vi "ME_acquire_21_HallSensor_LSchanB.vi"() -> ()   [LabVIEW 2015]
doc: "Use this template to build a producer/consumer design pattern. Use this template when you need to execute a process, such as data analysis, when a data source, such as a triggered acquisition, produces data at an uneven rate and you need to execute the process when the data becomes available."
uses:
  Mode.ctl
  oxford_driver/Oxford Drivers/BUSGEN.LLB/OxfordAddress.ctl
  <vilib>/Analysis/baseanly.llb/Mean (DBL).vi
  <vilib>/DAQmx/read.llb/DAQmx Read (Analog 1D DBL 1Chan NSamp).vi
  <vilib>/DAQmx/create/channels.llb/DAQmx Create Channel (AI-Voltage-Basic).vi
  <vilib>/DAQmx/configure/timing.llb/DAQmx Timing (Sample Clock).vi
  <vilib>/Utility/file.llb/Write Delimited Spreadsheet (DBL).vi
  <vilib>/DAQmx/miscellaneous.llb/DAQmx Fill In Error Info.vi
  <vilib>/express/express arith-compare/Formula/XNode/ExpressFormulaBlockNode.xnode
  <vilib>/Analysis/NI_AALBase.lvlib
panel:
  out "B lag":cluster{dbl[], dbl[]}(graph)
  out "T array":dbl[](array[numeric])
  out "Averaged I(T)":dbl[][](array[numeric])
  in  "Averaged P(T)":dbl[][](array[numeric])
  out "remaining elements 2":T1(array[cluster])
  out "Actual mean":dbl format="%0.6f"
  in  "Averaged dt":dbl[][](array[numeric])
  in  "Averaged P(B)":dbl[][](array[numeric])
  out "LockInR":dbl
  out "deltaUaux":dbl
  out "Hall Resistance (Ohm)":dbl caption="Actual AuxV" step=0.1
  in  "Stop":bool
  out "SaveSweep":bool=TRUE
  out "Measurement File_dn":path
  out "Measurement File_up":path
  out "Measurement File_average":path
  out "Actual Polarization":dbl
  in  "Reset IB?":bool
  in  "First?":bool
  in  "Save Period":dbl=1.0
  out "Averaged I(B)":dbl[][](array[numeric])
  out "P(uC/mm^2)":dbl[](array[numeric])
  in  "Sweep":bool
  out "Offset array":dbl[](array[numeric])
  in  "stop 2":bool
  in  "dB":dbl=0.005
  out "Actual B Field (T)":dbl
  out "Actual Temperature (K)":dbl
  out "Actual Current (pA)":dbl
  in  "Tab Control":T2(tab)
  in  "dt (K)":dbl=0.1
  in  "Max temperature (K)":dbl=20.0
  in  "Min Temperature (K)":dbl=4.5
  out "P(T)":cluster{"yi":dbl[], dbl[]}(graph)
  out "I(T)":cluster{dbl[], dbl[]}(graph)
  in  "Set temperature (K)":dbl=4.5
  in  "Temp Ramping Rate (K/min)":dbl=10.0
  in  "Heater Range":enum16{"Off", "Low", "Medium", "High"}(ring)
  in  "Heater On/Off":bool
  out "Setpoint Temperature (K)":dbl
  out "I(T) /Averaged/":cluster{"B array":dbl[], dbl[]}[](graph)
  out "P(T) /Averaged/":cluster{"B array":dbl[], dbl[]}[](graph)
  out "Up/Down 2":bool
  in  "Channel B/A":bool
  out "I(B) 3":cluster{dbl[], dbl[]}[](graph)
  out "I(B) /Averaged/":cluster{"B array":dbl[], dbl[]}[](graph)
  out "P(B) /Averaged/":cluster{"B array":dbl[], dbl[]}[](graph)
  out "P(B)":cluster{"yi":dbl[], dbl[]}(graph)
  in  "Set Field (T)":dbl
  in  "Go to Set":bool
  in  "Sweep Rate (T/min)":dbl=2.0 format="%.6f"
  in  "Field To Zero":bool
  out "Target Field":dbl
  in  "Min Field (T)":dbl
  in  "Max Field (T)":dbl=0.15
  in  "Threshold B (T)":dbl
  out "Up/Down":bool
  in  "Magnetic Field array (T)":dbl[](array[numeric])=[0.025, 0.05, 0.075, 0.1, 0.125, 0.15, 0.175, 0.2, 0.225, 0.25, 0.275, 0.3]
  in  "T Sweep Rate Array":dbl[](array[numeric])=[10.0, 20.0]
  in  "Max count array":i32[](array[numeric])=[2, 1, 0, 0, 0, 9, 10, 11, 12]
  in  "secs to wait":dbl=180.0
  out "Wait (s)":dbl
  in  "Directory":string
  out "Finished":bool=TRUE
  out "Step Rate":bool
  out "New":bool=TRUE
  in  "Temperature Array":dbl[](array[numeric])=[4.5, 5.0, 6.0, 7.0, 8.0, 9.0, 10.0, 11.0, 12.0]
  in  "Sweep Rate Array":dbl[](array[numeric])=[2.0, 1.0, 0.5, 0.1, 0.05, 9.0, 10.0, 11.0, 12.0]
  in  "Record ALL":bool
  in  "Max Countl":i32
  out "i":i32
  out "j":i32
  out "Step Temp":bool
  in  "FileName":string
  in  "Measure Noise":bool
  in  "Cycles":i32
  in  "maximum value":dbl=10.0 format="%0.2f"
  in  "minimum value":dbl=-10.0 format="%0.2f"
  in  "physical channels":tag="Dev1/ai1"
  out "PSD (pA/Hz^1/2) Peaks Removed":cluster{"f0":dbl, "df":dbl, "magnitude":dbl[]}(graph)
  out "PSD (pA/Hz^1/2)":cluster{"f0":dbl, "df":dbl, "magnitude":dbl[]}(graph)
  out "Current (pA) Filtered":waveform(dbl)(graph)
  out "Current (pA)":dbl[](graph)
  in  "Samples per channel":i32=1000
  in  "Rate":dbl=1000.0 format="%0.2f"
  in  "Cut-Off Frequency":dbl=100.0 caption="Lower Cut-Off"
  in  "Filter On":bool
  in  "Keithley (IV conv) averaging":i32=10
  in  "Lock_in_Amplifier":refnum<visa-resource-name>="GPIB0::5::INSTR"
  out "Dc offset":dbl
  in  "Calibrate":bool
  in  "IV converter":refnum<visa-resource-name>="GPIB0::20::INSTR"
  in  "Magnetic Field":refnum<visa-resource-name>="GPIB0::19::INSTR"
  out "Time Lag":dbl=0.0500025749206543
  in  "Lake Shore":refnum<visa-resource-name>="GPIB0::11::INSTR"
  in  "Temp Refresh (s)":dbl=0.1
  in  "Sampling rate (Hz)":dbl=10.0
  in  "Gain (V/A)":dbl=1000000000.0
  in  "Sample area (mm^2)":dbl=1.0
  out "Calibration Curve":cluster{dbl[], "Best Linear Fit":dbl[]}[](graph)=[{[0.0, 0.005, 0.01, 0.015, 0.02, 0.025, 0.03, 0.035, 0.04, 0.045, 0.05, 0.055, 0.06, 0.065, 0.07, 0.075, 0.08, 0.085, 0.09, 0.095, 0.1, 0.105, 0.11, 0.115, 0.12, 0.125, 0.13, 0.135, 0.14, 0.145, 0.15, 0.155, 0.16, 0.165, 0.17, 0.175, 0.18, 0.185, 0.19, 0.195, 0.2, 0.205, 0.21, 0.215, 0.22, 0.225, 0.23, 0.235, 0.24, 0.245, 0.25, 0.255, 0.26, 0.265, 0.27, 0.275, 0.28, 0.285, 0.29, 0.295, 0.3, 0.305, 0.31, 0.315, 0.32, 0.325, 0.33, 0.335, 0.34, 0.345, 0.35, 0.355, 0.36, 0.365, 0.37, 0.375, 0.38, 0.385, 0.39, 0.395, 0.4, 0.405, 0.41, 0.415, 0.42, 0.425, 0.43, 0.435, 0.44, 0.445, 0.45, 0.455, 0.46, 0.465, 0.47, 0.475, 0.48, 0.485, 0.49, 0.495, 0.5], "Best Linear Fit"=[-1.7e-06, 1.18e-05, 3.66e-05, 6.17e-05, 9.39e-05, 0.000122, 0.0001511, 0.0001781, 0.0002061, 0.0002355, 0.0002616, 0.0002895, 0.0003184, 0.0003446, 0.0003689, 0.0003958, 0.0004207, 0.0004464, 0.0004684, 0.0004953, 0.0005218, 0.0005459, 0.0005692, 0.0005897, 0.0006131, 0.0006347, 0.0006589, 0.0006834, 0.0007035, 0.0007249, 0.0007465, 0.000765, 0.0007858, 0.0008103, 0.0008302, 0.0008467, 0.000868, 0.0008855, 0.0009079, 0.0009248, 0.0009452, 0.0009633, 0.0009828, 0.0009992, 0.0010189, 0.0010338, 0.001054, 0.0010692, 0.0010858, 0.0011036, 0.0011162, 0.0011356, 0.0011502, 0.0011643, 0.0011834, 0.0011985, 0.0012131, 0.0012277, 0.0012423, 0.0012571, 0.0012691, 0.0012827, 0.0012976, 0.001313, 0.0013264, 0.0013388, 0.0013518, 0.0013638, 0.0013782, 0.0013909, 0.0014035, 0.0014175, 0.0014295, 0.0014407, 0.0014538, 0.0014641, 0.0014752, 0.0014861, 0.0014978, 0.0015081, 0.0015203, 0.001532, 0.0015422, 0.0015526, 0.001563, 0.0015754, 0.0015844, 0.0015955, 0.0016056, 0.001614, 0.0016239, 0.0016342, 0.0016457, 0.0016542, 0.0016635, 0.001674, 0.001681, 0.0016886, 0.0016986, 0.0017063, 0.0017155]}, {[0.0, 0.005, 0.01, 0.015, 0.02, 0.025, 0.03, 0.035, 0.04, 0.045, 0.05, 0.055, 0.06, 0.065, 0.07, 0.075, 0.08, 0.085, 0.09, 0.095, 0.1, 0.105, 0.11, 0.115, 0.12, 0.125, 0.13, 0.135, 0.14, 0.145, 0.15, 0.155, 0.16, 0.165, 0.17, 0.175, 0.18, 0.185, 0.19, 0.195, 0.2, 0.205, 0.21, 0.215, 0.22, 0.225, 0.23, 0.235, 0.24, 0.245, 0.25, 0.255, 0.26, 0.265, 0.27, 0.275, 0.28, 0.285, 0.29, 0.295, 0.3, 0.305, 0.31, 0.315, 0.32, 0.325, 0.33, 0.335, 0.34, 0.345, 0.35, 0.355, 0.36, 0.365, 0.37, 0.375, 0.38, 0.385, 0.39, 0.395, 0.4, 0.405, 0.41, 0.415, 0.42, 0.425, 0.43, 0.435, 0.44, 0.445, 0.45, 0.455, 0.46, 0.465, 0.47, 0.475, 0.48, 0.485, 0.49, 0.495, 0.5], "Best Linear Fit"=[-1.7e-06, 1.18e-05, 3.66e-05, 6.17e-05, 9.39e-05, 0.000122, 0.0001511, 0.0001781, 0.0002061, 0.0002355, 0.0002616, 0.0002895, 0.0003184, 0.0003446, 0.0003689, 0.0003958, 0.0004207, 0.0004464, 0.0004684, 0.0004953, 0.0005218, 0.0005459, 0.0005692, 0.0005897, 0.0006131, 0.0006347, 0.0006589, 0.0006834, 0.0007035, 0.0007249, 0.0007465, 0.000765, 0.0007858, 0.0008103, 0.0008302, 0.0008467, 0.000868, 0.0008855, 0.0009079, 0.0009248, 0.0009452, 0.0009633, 0.0009828, 0.0009992, 0.0010189, 0.0010338, 0.001054, 0.0010692, 0.0010858, 0.0011036, 0.0011162, 0.0011356, 0.0011502, 0.0011643, 0.0011834, 0.0011985, 0.0012131, 0.0012277, 0.0012423, 0.0012571, 0.0012691, 0.0012827, 0.0012976, 0.001313, 0.0013264, 0.0013388, 0.0013518, 0.0013638, 0.0013782, 0.0013909, 0.0014035, 0.0014175, 0.0014295, 0.0014407, 0.0014538, 0.0014641, 0.0014752, 0.0014861, 0.0014978, 0.0015081, 0.0015203, 0.001532, 0.0015422, 0.0015526, 0.001563, 0.0015754, 0.0015844, 0.0015955, 0.0016056, 0.001614, 0.0016239, 0.0016342, 0.0016457, 0.0016542, 0.0016635, 0.001674, 0.001681, 0.0016886, 0.0016986, 0.0017063, 0.0017155]}]
  in  "Offset?":bool
  in  "Magnet":bool=TRUE
  in  "Ramp":bool=TRUE
  in  "DaQ":bool
  in  "Moving average":i8=10
  in  "Sample Rate":dbl=1000.0
  in  "Number of Samples":i32=100
  in  "Physical Channel":tag="kartya/ai0"
  in  "Min Voltage":dbl=-5.0
  in  "Max Voltage":dbl=5.0
  in  "Terminal Configuration":i32(ring)=-1 items=["default"=-1, "RSE"=10083, "NRSE"=10078, "Differential"=10106, "Pseudodifferential"=12529]
  out "Confirm":bool
  in  "Dwell Time (ms)":u32=1000
  out "Calibration Curve Data":dbl[][](array[numeric])=[[0.0, 0.005, 0.01, 0.015, 0.02, 0.025, 0.03, 0.035, 0.04, 0.045, 0.05, 0.055, 0.06, 0.065, 0.07, 0.075, 0.08, 0.085, 0.09, 0.095, 0.1, 0.105, 0.11, 0.115, 0.12, 0.125, 0.13, 0.135, 0.14, 0.145, 0.15, 0.155, 0.16, 0.165, 0.17, 0.175, 0.18, 0.185, 0.19, 0.195, 0.2, 0.205, 0.21, 0.215, 0.22, 0.225, 0.23, 0.235, 0.24, 0.245, 0.25, 0.255, 0.26, 0.265, 0.27, 0.275, 0.28, 0.285, 0.29, 0.295, 0.3, 0.305, 0.31, 0.315, 0.32, 0.325, 0.33, 0.335, 0.34, 0.345, 0.35, 0.355, 0.36, 0.365, 0.37, 0.375, 0.38, 0.385, 0.39, 0.395, 0.4, 0.405, 0.41, 0.415, 0.42, 0.425, 0.43, 0.435, 0.44, 0.445, 0.45, 0.455, 0.46, 0.465, 0.47, 0.475, 0.48, 0.485, 0.49, 0.495, 0.5], [-1.7e-06, 1.18e-05, 3.66e-05, 6.17e-05, 9.39e-05, 0.000122, 0.0001511, 0.0001781, 0.0002061, 0.0002355, 0.0002616, 0.0002895, 0.0003184, 0.0003446, 0.0003689, 0.0003958, 0.0004207, 0.0004464, 0.0004684, 0.0004953, 0.0005218, 0.0005459, 0.0005692, 0.0005897, 0.0006131, 0.0006347, 0.0006589, 0.0006834, 0.0007035, 0.0007249, 0.0007465, 0.000765, 0.0007858, 0.0008103, 0.0008302, 0.0008467, 0.000868, 0.0008855, 0.0009079, 0.0009248, 0.0009452, 0.0009633, 0.0009828, 0.0009992, 0.0010189, 0.0010338, 0.001054, 0.0010692, 0.0010858, 0.0011036, 0.0011162, 0.0011356, 0.0011502, 0.0011643, 0.0011834, 0.0011985, 0.0012131, 0.0012277, 0.0012423, 0.0012571, 0.0012691, 0.0012827, 0.0012976, 0.001313, 0.0013264, 0.0013388, 0.0013518, 0.0013638, 0.0013782, 0.0013909, 0.0014035, 0.0014175, 0.0014295, 0.0014407, 0.0014538, 0.0014641, 0.0014752, 0.0014861, 0.0014978, 0.0015081, 0.0015203, 0.001532, 0.0015422, 0.0015526, 0.001563, 0.0015754, 0.0015844, 0.0015955, 0.0016056, 0.001614, 0.0016239, 0.0016342, 0.0016457, 0.0016542, 0.0016635, 0.001674, 0.001681, 0.0016886, 0.0016986, 0.0017063, 0.0017155]]
  in  "Start Field":dbl
  in  "Max Field":dbl=0.5 format="%#_13g"
  in  "Temp/Magnetic Field":bool
  out "index":i8
  out "Read?":bool
  out "Magnetic Field (T)":dbl[](array[numeric])
  out "Reset":bool
  out "Measured Current (pA)":dbl[](array[numeric])
  out "Elapsed Time (s)":dbl[](array[numeric])
  out "Start time":timestamp
  in  "Enum":T3=enum."Process"
  out "B array":dbl[](array[numeric])
  in  "dB (T)":dbl=0.0025
  in  "Counter":i8
  out "L magnet (H)":dbl
  out "R magnet (mOhm)":dbl
  out "Actual Current (R0)":dbl
  out "Nominal Field (T)":dbl
  out "Temperature array":dbl[](array[numeric])
  in  "New Measurement File":bool
  out "Measurement File":path
  out "refnum out":refnum<file>
  in  "Measuring":bool
  in  "Measure /Pause":bool
  in  "stop":bool
  # "DeltaForce"
  # "Discrete"
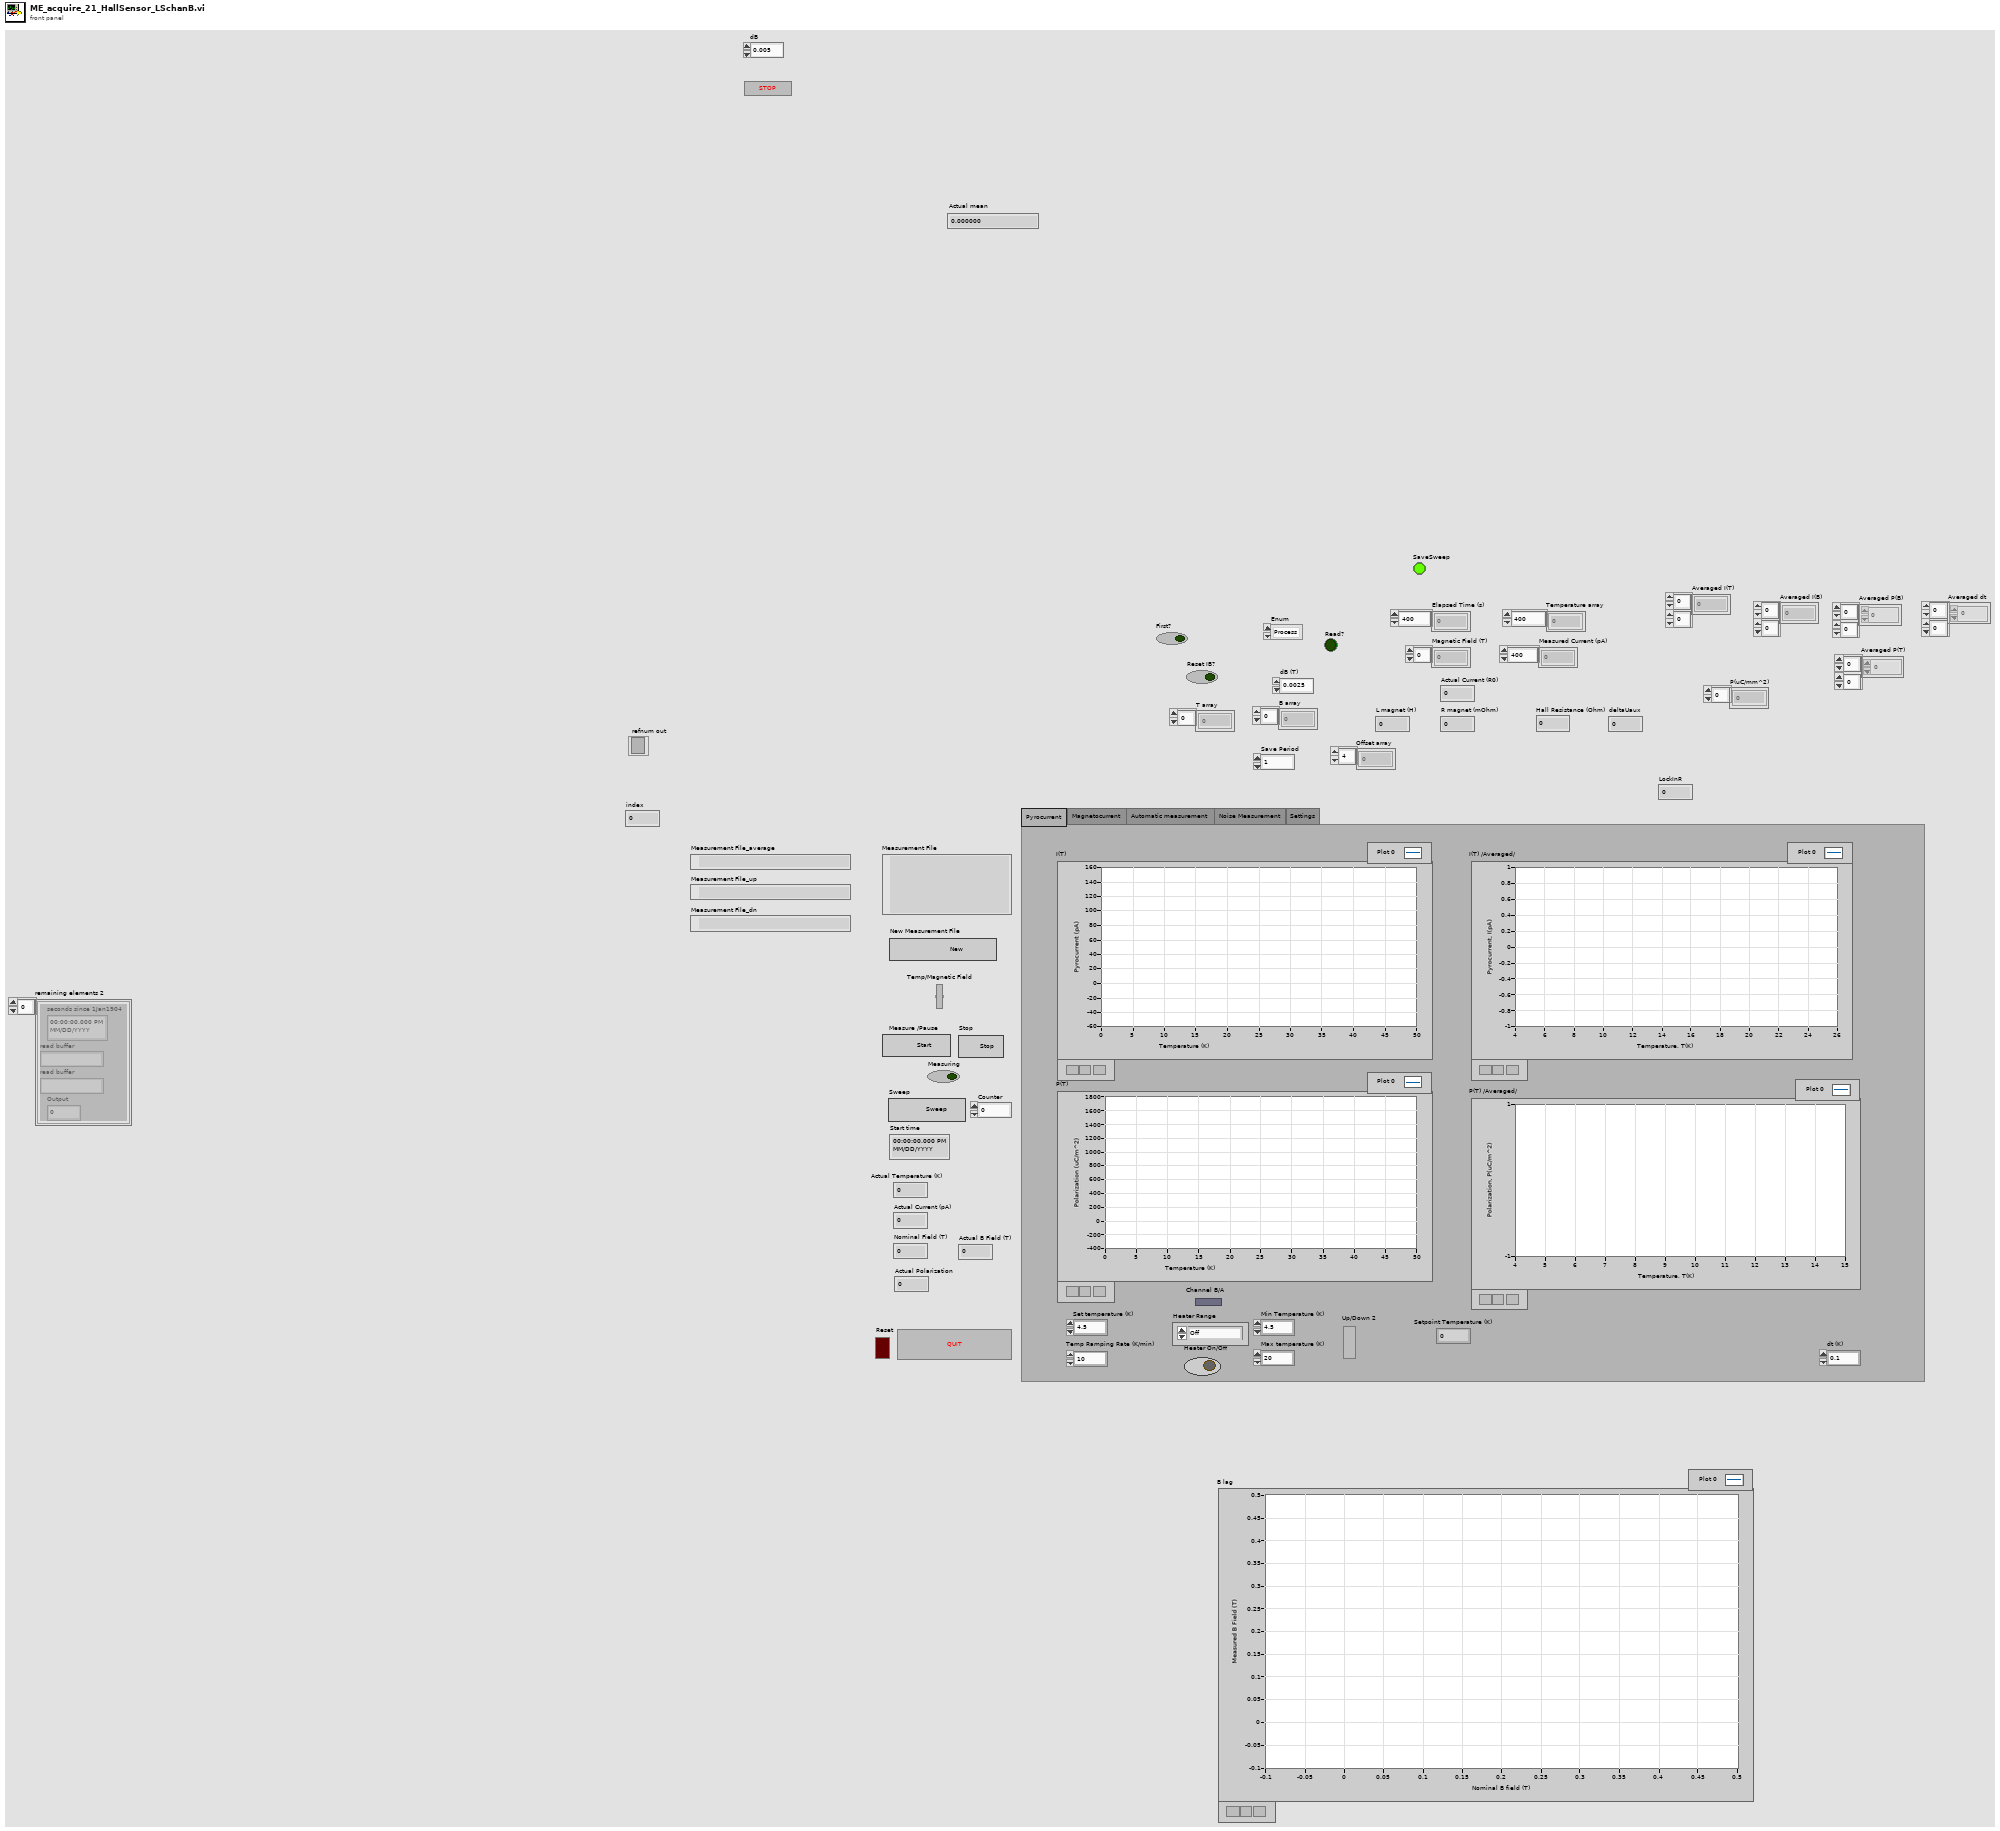
[diagram p1: front panel]
types:
  T1 = cluster{"seconds since 1Jan1904":timestamp, "read buffer":string, "read buffer":string, "Output":dbl}[]
  T2 = enum32{"Pyrocurrent", "Magnetocurrent", "Automatic measurement", "Noise Measurement", "Settings"}
  T3 = typedef "Mode.ctl" = enum16{"Offset", "Process", "Sweep", "StepOxford", "StepDelta", "Plot", "Save", "New", "Return", ""}
  T4 = cluster{"seconds since 1Jan1904":timestamp, "read buffer":string, "read buffer":string, "Output":dbl}
  T5 = enum16{"open", "replace", "create", "open or create", "replace or create", "replace or create with confirmation"}
  T6 = typedef "OxfordAddress.ctl" = cluster{"Com Port":i32, "ISOBUS Address":i32, "GPIB Address":i16, "Communication":enum16{"RS232", "ISOBUS", "GPIB", "Gateway"}}
  T7 = cluster{"B array":dbl[], "Averaged P(B) Out":dbl[]}
  T8 = cluster{"B array":dbl[], "BaselineSubtracted I(B)":dbl[]}
  T9 = cluster{"B array":dbl[], "Averaged P(B) Out":dbl[]}[]
  T10 = cluster{"B array":dbl[], "BaselineSubtracted I(B)":dbl[]}[]
  T11 = cluster{"T array":dbl[], "Averaged P(T) Out":dbl[]}
  T12 = cluster{"T array":dbl[], "Averaged I(B) out":dbl[]}
  T13 = cluster{"T array":dbl[], "Averaged P(T) Out":dbl[]}[]
  T14 = cluster{"T array":dbl[], "Averaged I(B) out":dbl[]}[]
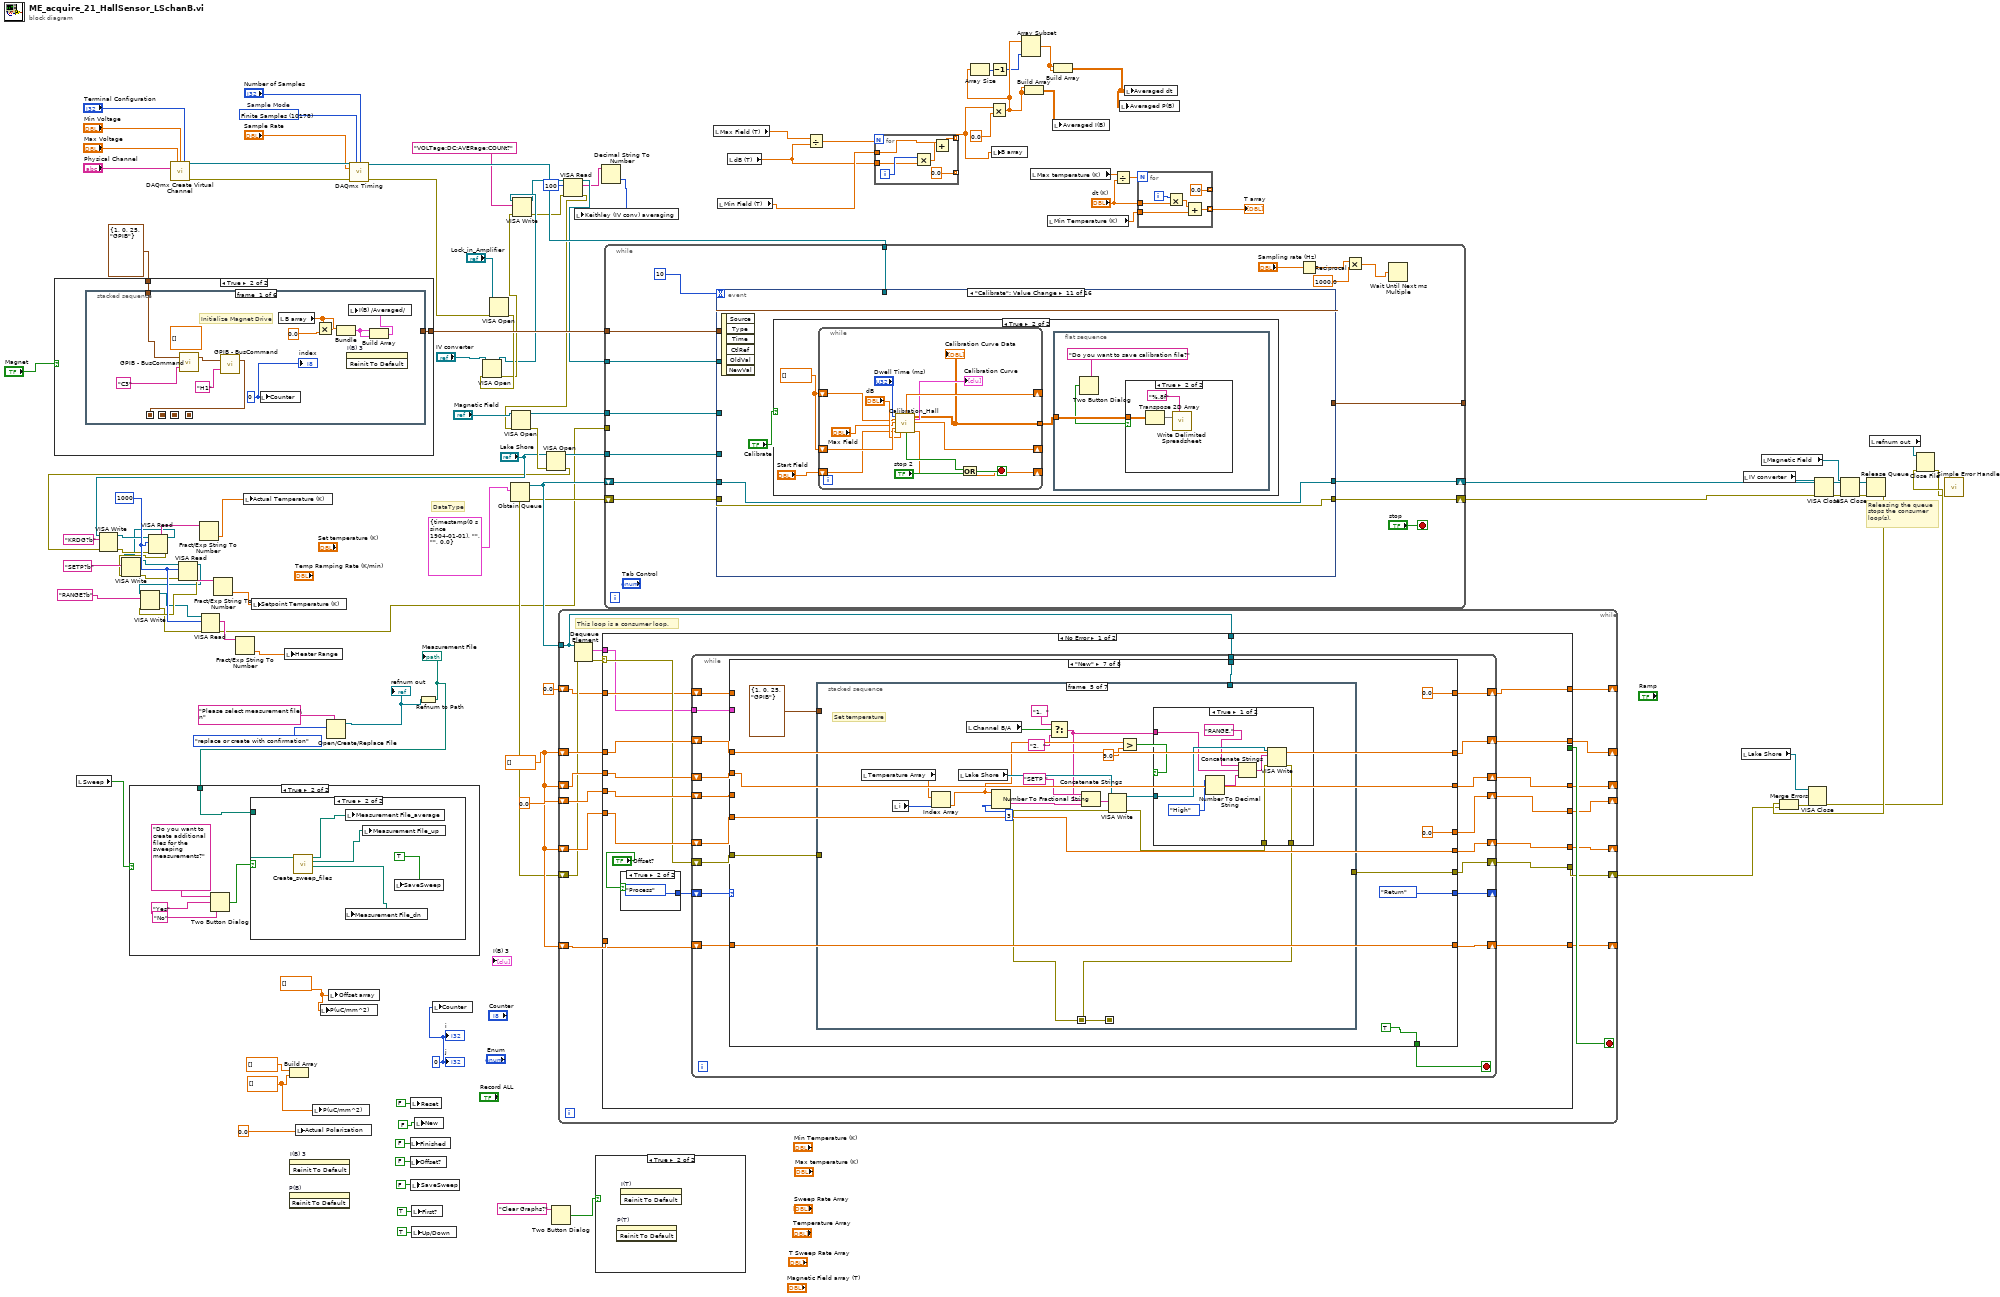
[diagram p0: block diagram]
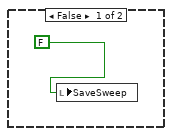
[diagram p4: hidden frame]
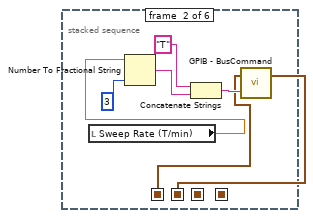
[diagram p6: hidden frame]
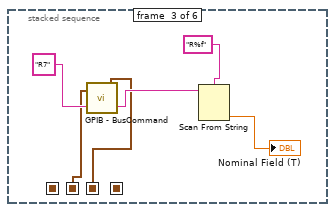
[diagram p7: hidden frame]
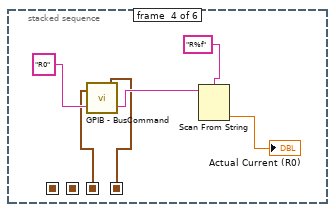
[diagram p8: hidden frame]
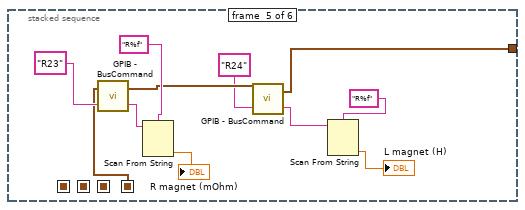
[diagram p9: hidden frame]
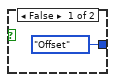
[diagram p11: hidden frame]
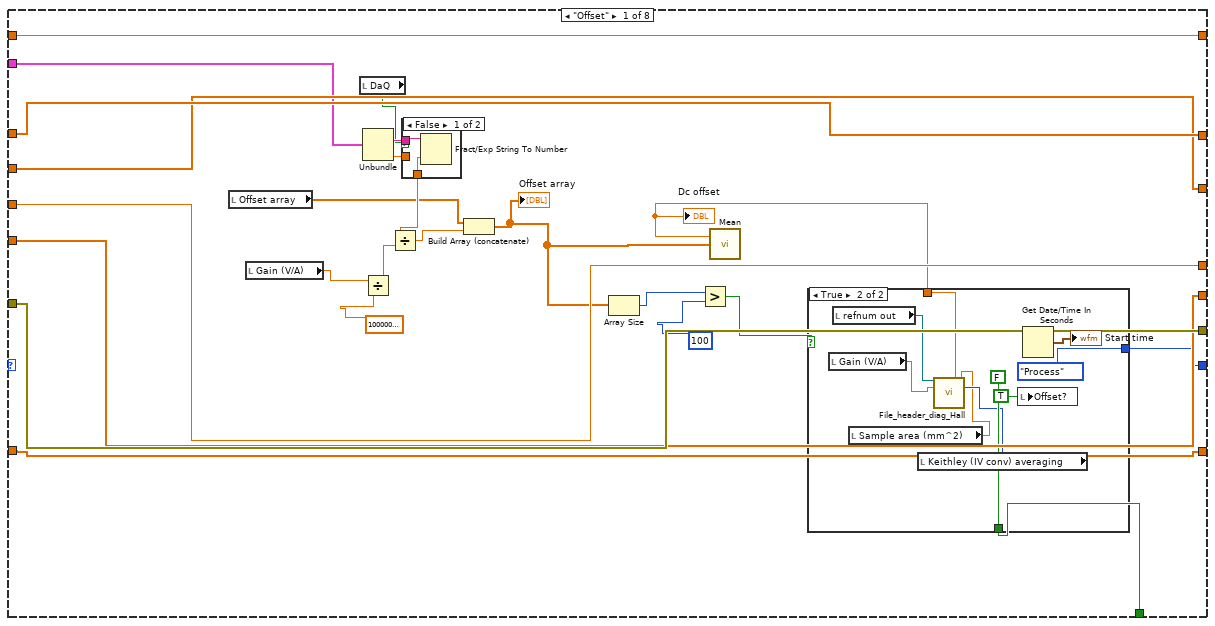
[diagram p12: hidden frame]
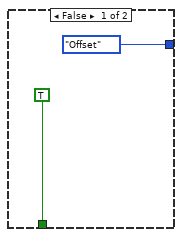
[diagram p14: hidden frame]
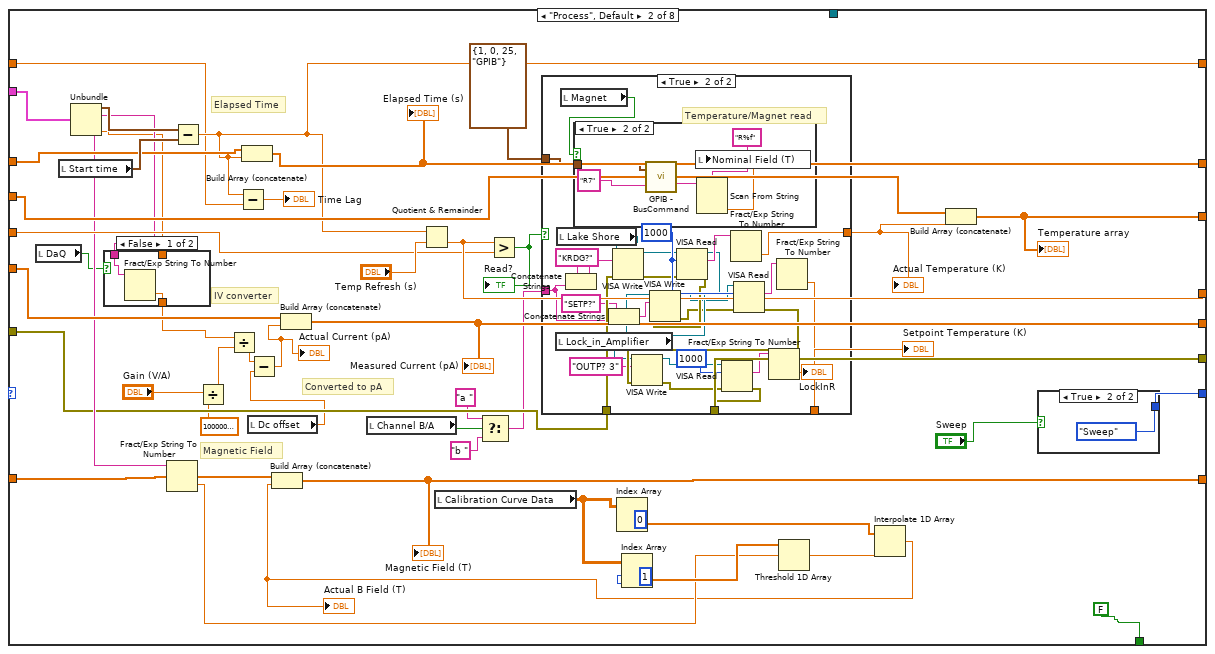
[diagram p15: hidden frame]
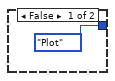
[diagram p17: hidden frame]
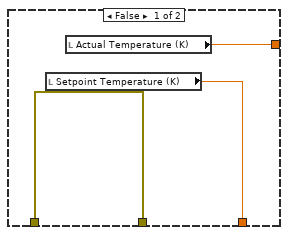
[diagram p18: hidden frame]
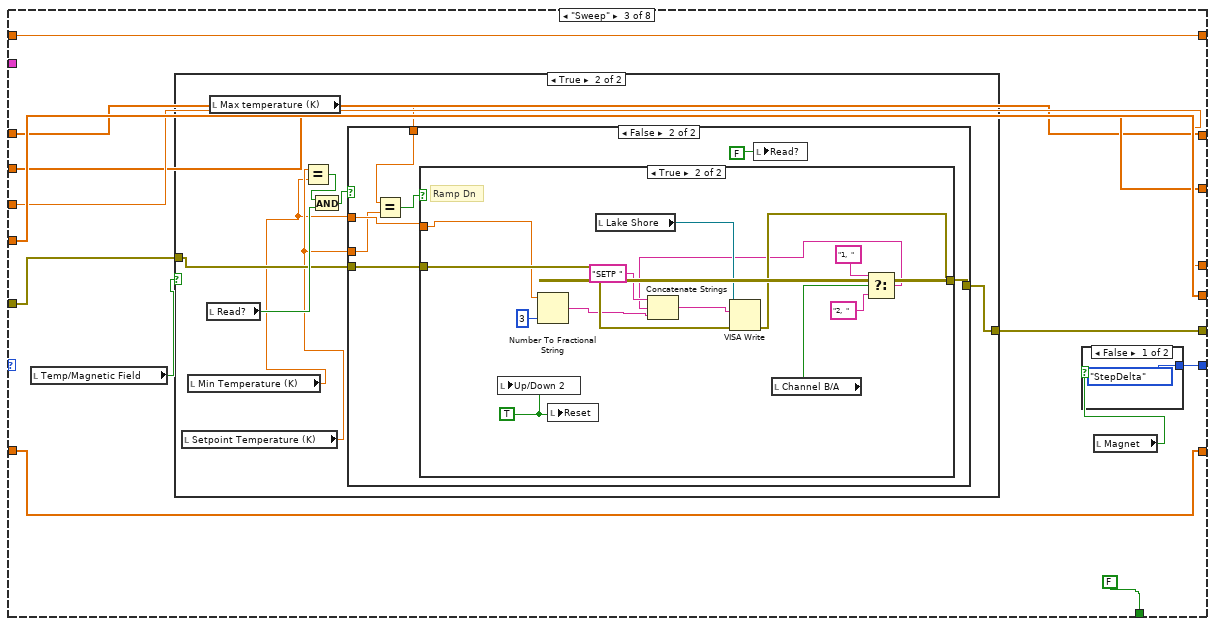
[diagram p20: hidden frame]
diagram:
  w27 = 10178 items=["Finite Samples"=10178, "Continuous Samples"=10123, "Hardware Timed Single Point"=12522]  # Sample Mode
  w54 = u32 1000 ("byte count")
  w65 = 0 ("j")
  w62 = dbl[] []
  w80 = dbl[] []
  w86 = dbl[] []
  # "DataType"
  # "Releasing the queue stops the consumer loop(s)."
  n1 = case shown="True" "Magnet" {
    tunnel: T6 {"Com Port"=1, "ISOBUS Address"=0, "GPIB Address"=25, "Communication"=enum."GPIB"} ("Address") -> [w110 w112]
    tunnel: [w110 w111] -> w92
    frame False {
    }
    frame True {
      n2 = stacked-sequence {
        seq-local: [w120 _ _ _ _ _] -> [_ w125 _ _ _ _]
        seq-local: [_ w124 _ _ _ _] -> [_ _ w132 _ _ _]
        seq-local: [_ _ w131 _ _ _] -> [_ _ _ w138 _ _]
        seq-local: [_ _ _ w137 _ _] -> [_ _ _ _ w149 _]
        tunnel: w112 -> [w122 _ _ _ _ _]
        tunnel: [_ _ _ _ w147 _] -> w111
        frame #0 {
          (unwired) dbl[][] []
          w118 = i8 0 ("Counter")
          # "Initialize Magnet Drive"
          n3 = call "GPIB - BusCommand.vi"("Command"="C3", "Address"=w122) -> ("Address(thru)"=w121:T6)  [unwired: 1 out]
          n4 = call "GPIB - BusCommand.vi"("Command"="H1", "Address"=w121) -> ("Address(thru)"=w120:T6)  [unwired: 1 out]
          n5 = local write "Counter"(w118) -> ()
          n6 = local read "B array"() -> (w116:dbl[])
          n7 = Multiply(x=w116, y=0.0) -> (x*y=w115:dbl[])
          n8 = Bundle("B array"=w116, w115) -> (w114:cluster{"B array":dbl[], dbl[]})  [unwired: 1 in]
          n9 = invoke on="I(B) 3" class="XYGraph (strict)" method="Reinit To Default"() -> ()  [unwired: 3 in, 3 out]
          n10 = Build Array(w114, w114) -> (w113:cluster{"B array":dbl[], dbl[]}[])
          n11 = local write "I(B) /Averaged/"(w113) -> ()
          "index" <- w118
        }
        frame #1 {
          n12 = local read "Sweep Rate (T/min)"() -> (w126:dbl)
          n13 = Number To Fractional String(number=w126, precision (6)=i16 3) -> (F-format string=w128:string)  [unwired: 2 in]
          n14 = Concatenate Strings("T" ("format string"), w128) -> (w127:string)
          n15 = call "GPIB - BusCommand.vi"("Command"=w127, "Address"=w125) -> ("Address(thru)"=w124:T6)  [unwired: 1 out]
        }
        frame #2 {
          n16 = call "GPIB - BusCommand.vi"("Command"="R7" ("format string"), "Address"=w132) -> ("Reply"=w136:string, "Address(thru)"=w131:T6)
          n17 = Scan From String(format string="R%f" ("remaining string"), input string=w136) -> (output 1=→"Nominal Field (T)":dbl)  [unwired: 3 in, 3 out]
        }
        frame #3 {
          n18 = call "GPIB - BusCommand.vi"("Command"="R0" ("format string"), "Address"=w138) -> ("Reply"=w142:string, "Address(thru)"=w137:T6)
          n19 = Scan From String(format string="R%f" ("remaining string"), input string=w142) -> (output 1=→"Actual Current (R0)":dbl)  [unwired: 3 in, 3 out]
        }
        frame #4 {
          n20 = call "GPIB - BusCommand.vi"("Command"="R23" ("format string"), "Address"=w149) -> ("Reply"=w153:string, "Address(thru)"=w148:T6)
          n21 = Scan From String(format string="R%f" ("remaining string"), input string=w153) -> (output 1=→"R magnet (mOhm)":dbl)  [unwired: 3 in, 3 out]
          n22 = call "GPIB - BusCommand.vi"("Command"="R24" ("format string"), "Address"=w148) -> ("Reply"=w145:string, "Address(thru)"=w147:T6)
          n23 = Scan From String(format string="R%f" ("remaining string"), input string=w145) -> (output 1=→"L magnet (H)":dbl)  [unwired: 3 in, 3 out]
        }
        frame #5 {
        }
      }
    }
  }
  n24 = local read "Sweep"() -> (w70:bool)
  n25 = call-poly <vilib>:"DAQmx Create Virtual Channel.vi"("maximum value"="Max Voltage", "minimum value"="Min Voltage", "input terminal configuration"="Terminal Configuration", "physical channels"="Physical Channel") -> ("task out"=w25:refnum<k21>, "error out"=w26:errorcluster)  [unwired: 10 in]
  n26 = Build Array(dbl[] [], w62) -> ()  [unwired: 1 out]
  n27 = invoke on="P(B)" class="XYGraph (strict)" method="Reinit To Default"() -> ()  [unwired: 3 in, 3 out]
  n28 = invoke on="I(B) 3" class="XYGraph (strict)" method="Reinit To Default"() -> ()  [unwired: 3 in, 3 out]
  n29 = local write "Actual Polarization"(0.0 ("Actual Polarization")) -> ()
  n30 = local write "P(uC/mm^2)"(w62) -> ()
  n31 = local write "P(uC/mm^2)"(w80) -> ()
  n32 = Open/Create/Replace File(prompt="Please select measurement file\n", operation (0:open)=T5."replace or create with confirmation") -> (refnum out=w89:refnum<file>)  [unwired: 4 in, 2 out]
  "refnum out" <- w89
  n33 = local write "Offset array"(w80) -> ()
  n34 = call-poly <vilib>:"DAQmx Timing.vi"("task/channels in"=w25, "sample mode"=w27, "samples per channel"="Number of Samples", "rate"="Sample Rate", "error in"=w26) -> ("task out"=w17:refnum<k21>, "error out"=w18:errorcluster)  [unwired: 9 in]
  n35 = local write "Finished"(FALSE ("Finished")) -> ()
  n36 = local write "Offset?"(FALSE ("Offset?")) -> ()
  n37 = local write "Reset"(FALSE ("Reset")) -> ()
  n38 = local write "SaveSweep"(FALSE ("SaveSweep")) -> ()
  n39 = local write "First?"(TRUE ("First?")) -> ()
  n40 = local write "Up/Down"(TRUE ("Up/Down")) -> ()
  n41 = local write "New"(FALSE ("New")) -> ()
  n42 = Refnum to Path(1:w89) -> (0:w69:path)
  "Measurement File" <- w69
  n43 = case shown="True" w70 {
    tunnel: w69 -> [_ w154]
    frame False {
    }
    frame True {
      n44 = Two Button Dialog(message="Do you want to create additional files for the sweeping measurements?" ("string"), 1:"No" ("F button name (\"Cancel\")"), 2:"Yes" ("T button name (\"OK\")")) -> (T button?=w156:bool)
      n45 = case shown="True" w156 {
        tunnel: w154 -> [_ w164]
        frame False {
          n46 = local write "SaveSweep"(FALSE ("SaveSweep")) -> ()
        }
        frame True {
          n47 = call "Create_sweep_files.vi"("Measurement File"=w164) -> ("Path 3"=w161:path, "Path 2"=w162:path, "Path"=w163:path)  [unwired: 8 in]
          n48 = local write "Measurement File_dn"(w161) -> ()
          n49 = local write "Measurement File_average"(w163) -> ()
          n50 = local write "Measurement File_up"(w162) -> ()
          n51 = local write "SaveSweep"(TRUE) -> ()
        }
      }
    }
  }
  n52 = local write "Counter"(w65) -> ()
  n53 = VISA Open(error in (no error)=w18, VISA resource name="Lock_in_Amplifier") -> (error out=w37:errorcluster)  [unwired: 3 in, 1 out]
  n54 = VISA Open(error in (no error)=w37, VISA resource name="IV converter") -> (VISA resource name=w14:refnum<visa-resource-name>, error out=w15:errorcluster)  [unwired: 3 in]
  n55 = Obtain Queue(element data type=T4 {"seconds since 1Jan1904"=timestamp(0 s since 1904-01-01), "read buffer"="", "read buffer"="", "Output"=0.0} ("output cluster")) -> (queue out=w109:refnum<queue>, error out=w84:errorcluster)  [unwired: 4 in, 1 out]
  n56 = VISA Write(VISA resource name=w14, write buffer="VOLTage:DC:AVERage:COUNt?", error in (no error)=w15) -> (VISA resource name out=w10:refnum<visa-resource-name>, error out=w12:errorcluster)  [unwired: 1 out]
  n57 = Two Button Dialog(message="Clear Graphs?") -> (T button?=w64:bool)  [unwired: 2 in]
  n58 = while {
    tunnel: w109 -> [w165]
    shift-right: [w178] -> _
    shift-left: w86 -> [w177]
    shift-right: [w176] -> _
    shift-left: w86 -> [w175]
    shift-right: [w174] -> _
    shift-left: w86 -> [w173]
    shift-right: [w172] -> _
    shift-left: 0.0 -> [w171]
    shift-right: [w170] -> _
    shift-left: w86 -> [w169]
    shift-right: [w179] -> w97
    shift-left: w84 -> [w168]
    shift-right: [w167] -> _
    shift-left: 0.0 -> [w166]
    stop <- w180 stop-if-true
    # "This loop is a consumer loop."
    n59 = Dequeue Element(queue=w165, error in (no error)=w168) -> (element=w181:T4, error out=w182:errorcluster)  [unwired: 1 in, 2 out]
    n60 = case shown="No Error" w182 {
      selector: w182 -> [w189 w956]
      tunnel: w181 -> [w183 _]
      tunnel: [_ TRUE] -> w180
      tunnel: [w188 w956] -> w179
      tunnel: [w199 w955] -> w178
      tunnel: w177 -> [w198 w955]
      tunnel: [w197 w952] -> w176
      tunnel: w175 -> [w196 w952]
      tunnel: [w195 w951] -> w174
      tunnel: w173 -> [w194 w951]
      tunnel: [w193 w953] -> w172
      tunnel: w171 -> [w192 w953]
      tunnel: [w191 w954] -> w170
      tunnel: w169 -> [w190 w954]
      tunnel: [w187 w950] -> w167
      tunnel: w166 -> [w186 w950]
      tunnel: w165 -> [w184 _]
      frame No Error {
        n61 = case shown="True" "Offset?" {
          tunnel: [Mode."Offset" ("Enum") Mode."Process" ("Enum")] -> w200
          frame False {
          }
          frame True {
          }
        }
        n62 = while {
          shift-right: [w209] -> _
          shift-left: w200 -> [w221]
          tunnel: w183 -> [w220]
          shift-right: [w219] -> w199
          shift-left: w198 -> [w218]
          shift-right: [w211] -> w191
          shift-left: w190 -> [w210]
          shift-right: [w213] -> w193
          shift-left: w192 -> [w212]
          shift-right: [w217] -> w197
          shift-left: w196 -> [w216]
          shift-right: [w207] -> w188
          shift-left: w189 -> [w208]
          shift-right: [w215] -> w195
          shift-left: w194 -> [w214]
          shift-right: [w205] -> w187
          shift-left: w186 -> [w204]
          tunnel: w184 -> [w203]
          stop <- w206 stop-if-true
          n63 = case shown="\"New\"" w221 {
            selector: w221 -> [_ _ _ _ _ _ _ w943]
            tunnel: w220 -> [w239 w306 _ _ _ _ _ _]
            tunnel: [w245 w303 w355 w497 w553 w626 w739 w948] -> w219
            tunnel: w218 -> [w245 w298 w355 w497 w553 w622 w739 w948]
            tunnel: [w240 w302 w358 w494 w555 w628 w737 w945] -> w217
            tunnel: w216 -> [w240 w301 w358 w494 w555 w623 w737 w945]
            tunnel: [w241 w300 w360 w492 w550 w629 w735 w942] -> w215
            tunnel: w214 -> [w241 w299 w360 w492 w550 w624 w735 w942]
            tunnel: [w243 w297 w357 w495 w551 w632 0.0 w946] -> w213
            tunnel: w212 -> [w243 w296 w357 w495 w551 w632 _ w946]
            tunnel: [w244 w293 w356 w496 w552 w627 w738 w947] -> w211
            tunnel: w210 -> [w244 w294 w356 w496 w552 w625 w738 w947]
            tunnel: [w228 w291 w353 Mode."Plot" ("Enum") Mode."Save" ("Enum") w633 Mode."Return" ("Enum") w943] -> w209
            tunnel: w208 -> [w242 w289 w362 w489 w558 w631 w731 w944]
            tunnel: [w242 w288 w361 w488 w558 w631 w730 w944] -> w207
            tunnel: [w224 FALSE FALSE FALSE FALSE w620 TRUE TRUE] -> w206
            tunnel: [w227 w285 w354 w490 w554 w630 0.0 w949] -> w205
            tunnel: w204 -> [w227 w284 w354 w490 w554 w630 _ w949]
            tunnel: w203 -> [_ _ _ _ _ _ w729 _]
            frame "Offset" {
              n64 = local read "Offset array"() -> (w233:dbl[])
              n65 = local read "Gain (V/A)"() -> (w237:dbl)
              n66 = local read "DaQ"() -> (w223:bool)
              n67 = Unbundle(w239) -> ("read buffer"=w226:string, "Output"=w222:dbl)  [unwired: 2 out]
              n68 = Divide(x=w237, y=1000000000000.0) -> (x/y=w235:dbl)
              n69 = case shown="False" w223 {
                tunnel: [w247 w248] -> w238
                tunnel: w226 -> [w246 _]
                tunnel: w222 -> [_ w248]
                frame False {
                  n70 = Fract/Exp String To Number(string=w246) -> (number=w247:dbl)  [unwired: 3 in, 1 out]
                }
                frame True {
                }
              }
              n71 = Divide(x=w238, y=w235) -> (x/y=w234:dbl)
              n72 = Build Array (concatenate)(w233, w234) -> (w229:dbl[])
              "Offset array" <- w229
              n73 = Array Size(array=w229) -> (size(s)=w232:i32)
              n74 = Greater?(x=w232, y=100) -> (0:w230:bool)
              n75 = call-poly <vilib>:"Mean.vi"("X"=w229) -> ("mean"=w225:dbl)  [unwired: 1 out]
              "Dc offset" <- w225
              n76 = case shown="True" w230 {
                tunnel: [Mode."Offset" ("Enum") Mode."Process" ("Enum")] -> w228
                tunnel: w225 -> [_ w255]
                tunnel: [TRUE FALSE] -> w224
                frame False {
                }
                frame True {
                  n77 = local read "Gain (V/A)"() -> (w256:dbl)
                  n78 = local read "refnum out"() -> (w257:refnum<file>)
                  n79 = local read "Sample area (mm^2)"() -> (w251:dbl)
                  n80 = local read "Keithley (IV conv) averaging"() -> (w252:i32)
                  n81 = call "File_header_diag_Hall.vi"("Byte Stream File in"=w257, "OFFSET"=w255, "Sample area"=w251, "Gain"=w256, "Averaging"=w252) -> ()  [unwired: 11 in]
                  n82 = local write "Offset?"(TRUE ("Offset?")) -> ()
                  n83 = Get Date/Time In Seconds() -> (seconds since 1Jan1904=→"Start time":timestamp)
                }
              }
            }
            frame "Process", Default {
              # "Converted to pA"
              # "Magnetic Field"
              # "IV converter"
              # "Elapsed Time"
              n84 = local read "DaQ"() -> (w274:bool)
              n85 = local read "Start time"() -> (w304:timestamp)
              n86 = Unbundle(w306) -> ("seconds since 1Jan1904"=w305:timestamp, "read buffer"=w275:string, "read buffer"=w290:string, "Output"=w272:dbl)
              n87 = case shown="False" w274 {
                tunnel: w275 -> [w310 _]
                tunnel: [w309 w311] -> w273
                tunnel: w272 -> [_ w311]
                frame False {
                  n88 = Fract/Exp String To Number(string=w310) -> (number=w309:dbl)  [unwired: 3 in, 1 out]
                }
                frame True {
                }
              }
              n89 = Fract/Exp String To Number(string=w290) -> (number=w267:dbl)  [unwired: 3 in, 1 out]
              n90 = Subtract(x=w305, y=w304) -> (x-y=w285:dbl)
              n91 = Divide(x="Gain (V/A)", y=1000000000000.0) -> (x/y=w283:dbl)
              n92 = Divide(x=w273, y=w283) -> (x/y=w280:dbl)
              n93 = Subtract(x=w285, y=w284) -> (x-y=→"Time Lag":dbl)
              n94 = Build Array (concatenate)(w298, w285) -> (w303:dbl[])
              "Elapsed Time (s)" <- w303
              n95 = local read "Dc offset"() -> (w278:dbl)
              n96 = Subtract(x=w280, y=w278) -> (x-y=w279:dbl)
              "Actual Current (pA)" <- w279
              n97 = Build Array (concatenate)(w301, w279) -> (w302:dbl[])
              "Measured Current (pA)" <- w302
              n98 = local read "Channel B/A"() -> (w262:bool)
              n99 = Quotient & Remainder(x=w285, y="Temp Refresh (s)") -> (floor(x/y)=w297:dbl)  [unwired: 1 out]
              n100 = local read "Calibration Curve Data"() -> (w269:dbl[][])
              n101 = Select(t="a " ("write buffer"), s=w262, f="b " ("write buffer")) -> (s? t:f=w260:string)
              n102 = Greater?(x=w297, y=w296) -> (0:w295:bool)
              "Read?" <- w295
              n103 = case shown="True" w295 {
                tunnel: [w315 w344] -> w292
                tunnel: w289 -> [w316 w343]
                tunnel: [w316 w324] -> w288
                tunnel: T6 {"Com Port"=1, "ISOBUS Address"=0, "GPIB Address"=25, "Communication"=enum."GPIB"} ("Address") -> [_ w342]
                tunnel: [w314 w339] -> w276
                tunnel: w260 -> [_ w318]
                frame False {
                  n104 = local read "Setpoint Temperature (K)"() -> (w314:dbl)
                  n105 = local read "Actual Temperature (K)"() -> (w315:dbl)
                }
                frame True {
                  w340 = u32 1000 ("byte count")
                  # "Temperature/Magnet read"
                  n106 = local read "Lock_in_Amplifier"() -> (w328:refnum<visa-resource-name>)
                  n107 = local read "Lake Shore"() -> (w341:refnum<visa-resource-name>)
                  n108 = local read "Magnet"() -> (w331:bool)
                  n109 = Concatenate Strings("KRDG?" ("write buffer"), w318) -> (w317:string)
                  n110 = case shown="True" w331 {
                    tunnel: w342 -> [_ w347]
                    frame False {
                    }
                    frame True {
                      n111 = call "GPIB - BusCommand.vi"("Command"="R7" ("format string"), "Address"=w347) -> ("Reply"=w348:string)  [unwired: 1 out]
                      n112 = Scan From String(format string="R%f" ("remaining string"), input string=w348) -> (output 1=w346:dbl)  [unwired: 3 in, 3 out]
                      n113 = local write "Nominal Field (T)"(w346) -> ()
                    }
                  }
                  n114 = Concatenate Strings("SETP?" ("write buffer"), w318) -> (w319:string)
                  n115 = VISA Write(VISA resource name=w341, write buffer=w317, error in (no error)=w343) -> (VISA resource name out=w338:refnum<visa-resource-name>, error out=w336:errorcluster)  [unwired: 1 out]
                  n116 = VISA Read(VISA resource name=w338, byte count=w340, error in (no error)=w336) -> (VISA resource name out=w337:refnum<visa-resource-name>, read buffer=w345:string, error out=w335:errorcluster)  [unwired: 1 out]
                  n117 = VISA Write(VISA resource name=w337, write buffer=w319, error in (no error)=w335) -> (VISA resource name out=w333:refnum<visa-resource-name>, error out=w334:errorcluster)  [unwired: 1 out]
                  n118 = Fract/Exp String To Number(string=w345) -> (number=w344:dbl)  [unwired: 3 in, 1 out]
                  n119 = VISA Read(VISA resource name=w333, byte count=w340, error in (no error)=w334) -> (read buffer=w332:string, error out=w330:errorcluster)  [unwired: 2 out]
                  n120 = VISA Write(VISA resource name=w328, write buffer="OUTP? 3", error in (no error)=w330) -> (VISA resource name out=w327:refnum<visa-resource-name>, error out=w329:errorcluster)  [unwired: 1 out]
                  n121 = VISA Read(VISA resource name=w327, byte count=u32 1000, error in (no error)=w329) -> (read buffer=w323:string, error out=w324:errorcluster)  [unwired: 2 out]
                  n122 = Fract/Exp String To Number(string=w323) -> (number=→"LockInR":dbl)  [unwired: 3 in, 1 out]
                  n123 = Fract/Exp String To Number(string=w332) -> (number=w339:dbl)  [unwired: 3 in, 1 out]
                }
              }
              "Actual Temperature (K)" <- w292
              "Setpoint Temperature (K)" <- w276
              n124 = Index Array(array=w269, index (row)=0) -> (element=w265:dbl[])  [unwired: 1 in]
              n125 = Index Array(array=w269, index (row)=1 ("index (col)")) -> (element=w268:dbl[])  [unwired: 1 in]
              n126 = Threshold 1D Array(2:w267, 3:w268) -> (0:w266:dbl)  [unwired: 1 in]
              n127 = Interpolate 1D Array(1:w266, 2:w265) -> (0:w264:dbl)
              "Actual B Field (T)" <- w264
              n128 = Build Array (concatenate)(w299, w264) -> (w300:dbl[])
              "Magnetic Field (T)" <- w300
              n129 = Build Array (concatenate)(w294, w292) -> (w293:dbl[])
              "Temperature array" <- w293
              n130 = case shown="True" "Sweep" {
                tunnel: [Mode."Plot" ("Enum") Mode."Sweep" ("Enum")] -> w291
                frame False {
                }
                frame True {
                }
              }
            }
            frame "Sweep" {
              n131 = local read "Temp/Magnetic Field"() -> (w352:bool)
              n132 = case shown="True" w352 {
                tunnel: w362 -> [w371 w428]
                tunnel: [w370 w427] -> w361
                frame False {
                  n133 = local read "Nominal Field (T)"() -> (w366:dbl)
                  n134 = local read "Min Field (T)"() -> (w365:dbl)
                  n135 = local read "Max Field (T)"() -> (w372:dbl)
                  n136 = local read "Read?"() -> (w369:bool)
                  n137 = Greater Or Equal?(x=w365, y=w366) -> (x >= y?=w368:bool)
                  n138 = Compound Arithmetic op=AND(w368, w369) -> (w367:bool)
                  n139 = case shown="False" w367 {
                    tunnel: [w375 w411] -> w370
                    tunnel: w372 -> [w373 w410]
                    tunnel: w365 -> [_ w409]
                    tunnel: w366 -> [_ w407]
                    tunnel: w371 -> [w376 w406]
                    frame True {
                      # "Ramp Up"
                      n140 = case shown="True" "First?" {
                        tunnel: [TRUE ("Save") FALSE ("Save")] -> w379
                        tunnel: [w398 w402] -> w378
                        frame False {
                          n141 = local read "Counter"() -> (w401:i8)
                          n142 = local write "Actual Polarization"(0.0 ("Actual Polarization")) -> ()
                          n143 = Increment(x=w401) -> (x+1=w398:i8)
                          n144 = local write "Counter"(w398) -> ()
                        }
                        frame True {
                          n145 = local read "Counter"() -> (w402:i8)
                          n146 = local write "First?"(FALSE ("First?")) -> ()
                        }
                      }
                      "Reset" <- w379
                      n147 = local write "Read?"(FALSE ("Read?")) -> ()
                      n148 = local read "Record ALL"() -> (w374:bool)
                      n149 = case shown="True" w374 {
                        tunnel: w378 -> [_ w386]
                        tunnel: [FALSE w384] -> w377
                        frame False {
                        }
                        frame True {
                          n150 = Greater?(x=w386, y="Max Countl") -> (0:w384:bool)
                        }
                      }
                      n151 = case shown="True" w377 {
                        tunnel: w376 -> [w390 w397]
                        tunnel: [w389 w397] -> w375
                        tunnel: w373 -> [w388 _]
                        frame False {
                          n152 = local read "Magnet"() -> (w387:bool)
                          n153 = case shown="True" w387 {
                            tunnel: w390 -> [w391 w394]
                            tunnel: [w391 w393] -> w389
                            tunnel: w388 -> [_ w392]
                            frame False {
                            }
                            frame True {
                              n154 = call "Set_B.vi"("error in (no error)"=w394, "address string"="25", "Set Field (T)"=w392) -> ("error out"=w393:errorcluster)  [unwired: 8 in]
                            }
                          }
                          "Target Field" <- w388
                        }
                        frame True {
                          "New" <- TRUE
                        }
                      }
                      "Up/Down" <- FALSE ("Up/Down")
                    }
                    frame False {
                      n155 = Less Or Equal?(x=w410, y=w407) -> (x <= y?=w408:bool)
                      n156 = case shown="True" w408 {
                        tunnel: [w412 w416] -> w411
                        tunnel: w409 -> [_ w414]
                        tunnel: w406 -> [w412 w417]
                        frame False {
                        }
                        frame True {
                          # "Resetting at the end of every cycle"
                          # "Ramp Dn"
                          n157 = local write "Up/Down"(TRUE ("Up/Down")) -> ()
                          n158 = local read "Magnet"() -> (w413:bool)
                          n159 = local write "Target Field"(w414) -> ()
                          n160 = local write "Reset"(TRUE ("Reset")) -> ()
                          n161 = case shown="True" w413 {
                            tunnel: w417 -> [w419 w422]
                            tunnel: [w419 w421] -> w416
                            tunnel: w414 -> [_ w420]
                            frame False {
                            }
                            frame True {
                              n162 = call "Set_B.vi"("error in (no error)"=w422, "address string"="25", "Set Field (T)"=w420) -> ("error out"=w421:errorcluster)  [unwired: 8 in]
                            }
                          }
                        }
                      }
                      n163 = local write "Read?"(FALSE ("Read?")) -> ()
                    }
                  }
                }
                frame True {
                  n164 = local read "Setpoint Temperature (K)"() -> (w426:dbl)
                  n165 = local read "Min Temperature (K)"() -> (w425:dbl)
                  n166 = local read "Read?"() -> (w431:bool)
                  n167 = local read "Max temperature (K)"() -> (w424:dbl)
                  n168 = Equal?(x=w426, y=w425) -> (x = y?=w429:bool)
                  n169 = And(x=w429, y=w431) -> (x .and. y?=w430:bool)
                  n170 = case shown="False" w430 {
                    tunnel: [w437 w473] -> w427
                    tunnel: w424 -> [w445 w472]
                    tunnel: w425 -> [_ w471]
                    tunnel: w426 -> [_ w469]
                    tunnel: w428 -> [w438 w468]
                    frame True {
                      # "Ramp Up"
                      n171 = local read "First?"() -> (w448:bool)
                      n172 = case shown="False" w448 {
                        tunnel: [TRUE ("Save") FALSE ("Save")] -> w440
                        tunnel: [w460 w466] -> w443
                        frame False {
                          n173 = local read "Counter"() -> (w463:i8)
                          n174 = local write "Actual Polarization"(0.0 ("Actual Polarization")) -> ()
                          n175 = Increment(x=w463) -> (x+1=w460:i8)
                          n176 = local write "Counter"(w460) -> ()
                        }
                        frame True {
                          n177 = local read "Counter"() -> (w466:i8)
                          n178 = local write "First?"(FALSE ("First?")) -> ()
                        }
                      }
                      n179 = local write "Read?"(FALSE ("Read?")) -> ()
                      n180 = Number To Fractional String(number=w445, precision (6)=i16 3) -> (F-format string=w433:string)  [unwired: 2 in]
                      n181 = local read "Record ALL"() -> (w444:bool)
                      n182 = local read "Channel B/A"() -> (w434:bool)
                      n183 = case shown="True" w444 {
                        tunnel: w443 -> [_ w459]
                        tunnel: [FALSE w458] -> w441
                        frame False {
                        }
                        frame True {
                          n184 = local read "Max Countl"() -> (w457:i32)
                          n185 = Greater?(x=w459, y=w457) -> (0:w458:bool)
                        }
                      }
                      n186 = local write "Reset"(w440) -> ()
                      n187 = Select(t="1,  " ("write buffer"), s=w434, f="2,  " ("write buffer")) -> (s? t:f=w432:string)
                      n188 = Concatenate Strings("SETP " ("write buffer"), w432, w433) -> (w439:string)
                      n189 = case shown="True" w441 {
                        tunnel: w439 -> [w453 _]
                        tunnel: w438 -> [w451 w454]
                        tunnel: [w450 w454] -> w437
                        frame False {
                          n190 = local read "Lake Shore"() -> (w452:refnum<visa-resource-name>)
                          n191 = VISA Write(VISA resource name=w452, write buffer=w453, error in (no error)=w451) -> (error out=w450:errorcluster)  [unwired: 2 out]
                        }
                        frame True {
                          n192 = local write "New"(TRUE ("New")) -> ()
                        }
                      }
                      "Up/Down 2" <- FALSE ("Up/Down")
                    }
                    frame False {
                      n193 = Equal?(x=w472, y=w469) -> (x = y?=w470:bool)
                      n194 = case shown="True" w470 {
                        tunnel: [w474 w485] -> w473
                        tunnel: w471 -> [_ w484]
                        tunnel: w468 -> [w474 w486]
                        frame False {
                        }
                        frame True {
                          w482 = TRUE ("Reset")
                          # "Ramp Dn"
                          n195 = local write "Up/Down 2"(w482) -> ()
                          n196 = Number To Fractional String(number=w484, precision (6)=i16 3) -> (F-format string=w477:string)  [unwired: 2 in]
                          n197 = local write "Reset"(w482) -> ()
                          n198 = local read "Lake Shore"() -> (w483:refnum<visa-resource-name>)
                          n199 = local read "Channel B/A"() -> (w478:bool)
                          n200 = Select(t="1,  " ("write buffer"), s=w478, f="2,  " ("write buffer")) -> (s? t:f=w476:string)
                          n201 = Concatenate Strings("SETP " ("write buffer"), w476, w477) -> (w475:string)
                          n202 = VISA Write(VISA resource name=w483, write buffer=w475, error in (no error)=w486) -> (error out=w485:errorcluster)  [unwired: 2 out]
                        }
                      }
                      n203 = local write "Read?"(FALSE ("Read?")) -> ()
                    }
                  }
                }
              }
              n204 = local read "Magnet"() -> (w351:bool)
              n205 = case shown="False" w351 {
                tunnel: [Mode."StepDelta" ("Enum") Mode."Plot" ("Enum")] -> w353
                frame False {
                }
                frame True {
                }
              }
            }
            frame "StepDelta" {
              n206 = flat-sequence {
                tunnel: w489 -> [w504]
                tunnel: [w503] -> w488
                frame #0 {
                  # "Check if it is time to step Field"
                  n207 = local read "Sweep Rate (T/min)"() -> (w505:dbl)
                  n208 = local read "Time Lag"() -> (w501:dbl)
                  n209 = xnode "Sweep Delay"("SweepRate"=w505, "Resolution"=0.001 ("Voltage Step (V)")) -> ("Result"=w502:dbl)  [unwired: 2 in, 1 out]
                  n210 = Divide(x=w501, y=w502) -> (x/y=w499:dbl)
                  n211 = Multiply(x=0.001 ("y"), y=w499) -> (x*y=w498:dbl)
                  "deltaUaux" <- w498
                  n212 = stacked-sequence {
                    tunnel: w504 -> [_ w516]
                    tunnel: [_ w515] -> w503
                    tunnel: w498 -> [w510 _]
                    frame #0 {
                      n213 = local read "Hall Resistance (Ohm)"() -> (w513:dbl)
                      n214 = local read "Up/Down"() -> (w514:bool)
                      n215 = Add(x=w513, y=w510) -> (x+y=w512:dbl)
                      n216 = Subtract(x=w513, y=w510) -> (x-y=w511:dbl)
                      n217 = local read "Calibration Curve Data"() -> (w509:dbl[][])
                      n218 = Select(t=w511, s=w514, f=w512) -> (s? t:f=w507:dbl)
                      "Hall Resistance (Ohm)" <- w507
                      n219 = call "HallR_to_B.vi"("Measured R(Ohm)"=w507, "Calibration Curve Data"=w509) -> ("Interpolated B value"=w508:dbl)  [unwired: 9 in]
                      n220 = local write "Nominal Field (T)"(w508) -> ()
                    }
                    frame #1 {
                      n221 = local read "Hall Resistance (Ohm)"() -> (w521:dbl)
                      n222 = local read "Lock_in_Amplifier"() -> (w517:refnum<visa-resource-name>)
                      n223 = Format Into String(w521) -> (resulting string=w520:string)  [unwired: 3 in, 1 out]
                      n224 = Concatenate Strings("AUXV 1,", w520) -> (w518:string)
                      n225 = VISA Write(VISA resource name=w517, write buffer=w518, error in (no error)=w516) -> (error out=w515:errorcluster)  [unwired: 2 out]
                    }
                  }
                }
              }
            }
            frame "Plot" {
              # "dI"
              n226 = local read "Nominal Field (T)"() -> (w541:dbl)
              n227 = local read "Actual B Field (T)"() -> (w540:dbl)
              n228 = local read "P(uC/mm^2)"() -> (w543:dbl[])
              n229 = local read "B lag"() -> (w536:cluster{dbl[], dbl[]})
              n230 = local read "Actual Polarization"() -> (w542:dbl)
              n231 = Unbundle(w536) -> (w535:dbl[], w534:dbl[])
              n232 = Build Array (concatenate)(w534, w540) -> (w538:dbl[])
              n233 = Build Array (concatenate)(w535, w541) -> (w539:dbl[])
              n234 = local read "Actual Current (pA)"() -> (w544:dbl)
              n235 = local read "Time Lag"() -> (w556:dbl)
              n236 = Bundle(w539, w538) -> (→"B lag":cluster{dbl[], dbl[]})  [unwired: 1 in]
              n237 = Multiply(x=w544, y=w556) -> (x*y=w548:dbl)
              n238 = Divide(x=w548, y="Sample area (mm^2)") -> (x/y=w547:dbl)
              n239 = Add(x=w547, y=w542) -> (x+y=w546:dbl)
              "Actual Polarization" <- w546
              n240 = local read "Temp/Magnetic Field"() -> (w557:bool)
              n241 = Build Array (concatenate)(w543, w546) -> (→"P(uC/mm^2)":dbl[])
              n242 = case shown="False" w557 {
                tunnel: w554 -> [_ w617]
                tunnel: w551 -> [_ w599]
                tunnel: w546 -> [w564 w600]
                frame False {
                  # "Magnetic Field plotting"
                  n243 = local read "Up/Down"() -> (w569:bool)
                  n244 = case shown="False" w569 {
                    frame True {
                      # "Down"
                      n245 = local read "I(B) 3"() -> (w579:cluster{dbl[], dbl[]}[])
                      n246 = local read "I(B) 3"() -> (w583:cluster{dbl[], dbl[]}[])
                      n247 = Index Array(array=w579, index=1) -> (element=w577:cluster{dbl[], dbl[]})
                      n248 = Unbundle(w577) -> (w576:dbl[], w575:dbl[])
                      n249 = Index Array(array=w583, index=i8 0 ("t")) -> (element=w580:cluster{dbl[], dbl[]})
                      n250 = local read "Actual Current (pA)"() -> (w570:dbl)
                      n251 = local read "Actual B Field (T)"() -> (w572:dbl)
                      n252 = Build Array (concatenate)(w576, w572) -> (w574:dbl[])
                      n253 = Build Array (concatenate)(w575, w570) -> (w573:dbl[])
                      n254 = Bundle(w574, w573) -> (w571:cluster{dbl[], dbl[]})  [unwired: 1 in]
                      n255 = Build Array(w580, w571) -> (w581:cluster{dbl[], dbl[]}[])
                      n256 = local write "I(B) 3"(w581) -> ()
                    }
                    frame False {
                      # "Up"
                      n257 = local read "I(B) 3"() -> (w595:cluster{dbl[], dbl[]}[])
                      n258 = local read "I(B) 3"() -> (w597:cluster{dbl[], dbl[]}[])
                      n259 = Index Array(array=w595, index=0) -> (element=w593:cluster{dbl[], dbl[]})
                      n260 = Unbundle(w593) -> (w592:dbl[], w591:dbl[])
                      n261 = Index Array(array=w597, index=i8 1 ("t")) -> (element=w586:cluster{dbl[], dbl[]})
                      n262 = local read "Actual B Field (T)"() -> (w587:dbl)
                      n263 = Build Array (concatenate)(w592, w587) -> (w590:dbl[])
                      n264 = local read "Actual Current (pA)"() -> (w584:dbl)
                      n265 = Build Array (concatenate)(w591, w584) -> (w589:dbl[])
                      n266 = Bundle(w590, w589) -> (w588:cluster{dbl[], dbl[]})  [unwired: 1 in]
                      n267 = Build Array(w588, w586) -> (w585:cluster{dbl[], dbl[]}[])
                      n268 = local write "I(B) 3"(w585) -> ()
                    }
                  }
                  n269 = local read "Actual B Field (T)"() -> (w566:dbl)
                  n270 = local read "P(B)"() -> (w568:cluster{"yi":dbl[], dbl[]})
                  n271 = Unbundle(w568) -> ("yi"=w567:dbl[], w565:dbl[])
                  n272 = Build Array (concatenate)(w567, w566) -> (w563:dbl[])
                  n273 = Build Array (concatenate)(w565, w564) -> (w562:dbl[])
                  n274 = Bundle(w563, w562) -> (→"P(B)":cluster{dbl[], dbl[]})  [unwired: 1 in]
                }
                frame True {
                  # "Temperature plotting"
                  n275 = Quotient & Remainder(x=w617, y="Save Period") -> (x-y*floor(x/y)=w598:dbl)  [unwired: 1 out]
                  n276 = Greater?(x=w599, y=w598) -> (0:w615:bool)
                  n277 = local read "Actual Temperature (K)"() -> (w602:dbl)
                  n278 = local read "Actual Current (pA)"() -> (w608:dbl)
                  n279 = local read "P(T)"() -> (w604:cluster{"yi":dbl[], dbl[]})
                  n280 = local read "I(T)"() -> (w614:cluster{dbl[], dbl[]})
                  n281 = case shown="True" w615 {
                    frame False {
                    }
                    frame True {
                      n282 = local write "Reset"(TRUE) -> ()
                    }
                  }
                  n283 = Unbundle(w604) -> ("yi"=w605:dbl[], w601:dbl[])
                  n284 = Unbundle(w614) -> (w612:dbl[], w611:dbl[])
                  n285 = Build Array (concatenate)(w605, w602) -> (w606:dbl[])
                  n286 = Build Array (concatenate)(w601, w600) -> (w607:dbl[])
                  n287 = Build Array (concatenate)(w612, w602) -> (w610:dbl[])
                  n288 = Build Array (concatenate)(w611, w608) -> (w609:dbl[])
                  n289 = Bundle(w610, w609) -> (→"I(T)":cluster{dbl[], dbl[]})  [unwired: 1 in]
                  n290 = Bundle(w606, w607) -> (→"P(T)":cluster{dbl[], dbl[]})  [unwired: 1 in]
                }
              }
            }
            frame "Save" {
              n291 = local read "Reset"() -> (w619:bool)
              n292 = case shown="True" w619 {
                tunnel: w624 -> [w641 w643]
                tunnel: [w641 w646] -> w629
                tunnel: w623 -> [w640 w644]
                tunnel: [w640 w646] -> w628
                tunnel: w625 -> [w639 w645]
                tunnel: [w639 w646] -> w627
                tunnel: [w638 w646] -> w626
                tunnel: w622 -> [w638 w642]
                frame False {
                }
                frame True {
                  n293 = stacked-sequence {
                    tunnel: [_ _ w728] -> w646
                    tunnel: w645 -> [_ w717 _]
                    tunnel: w644 -> [w649 w715 _]
                    tunnel: w643 -> [w650 w716 _]
                    tunnel: w642 -> [w648 w713 _]
                    frame #0 {
                      n294 = local read "Temp/Magnetic Field"() -> (w647:bool)
                      n295 = case shown="True" w647 {
                        tunnel: w650 -> [w677 w704]
                        tunnel: w649 -> [w676 w703]
                        tunnel: w648 -> [w667 w694]
                        frame False {
                          n296 = local read "B array"() -> (w661:dbl[])
                          n297 = local read "Counter"() -> (w675:i8)
                          n298 = local read "Averaged I(B)"() -> (w652:dbl[][])
                          n299 = local read "Up/Down"() -> (w678:bool)
                          n300 = local read "Sample area (mm^2)"() -> (w657:dbl)
                          n301 = call "Average_IBP_curves_baseline.vi"("I in"=w676, "Averaged P(B) In"="Averaged P(B)", "Counter"=w675, "B0"="Threshold B (T)", "Averaged I(B) In"=w652, "t in"=w667, "B in"=w677, "Averaged dt in"="Averaged dt", "Up/Down"=w678, "Sample area(mm^2)"=w657, "B array"=w661) -> ("Averaged dt Out"=w664:dbl[][], "Averaged P(B) Out"=w653:dbl[][], "BaselineSubtracted I(B)"=w651:dbl[][])  [unwired: 1 in, 1 out]
                          "Averaged I(B)" <- w651
                          n302 = Index Array(array=w653, index (row)=0 ("disabled index (col)")) -> (element=w662:dbl[])  [unwired: 1 in]
                          n303 = Index Array(array=w653, index (row)=1 ("disabled index (col)")) -> (element=w663:dbl[])  [unwired: 1 in]
                          n304 = Index Array(array=w651, index (row)=0 ("disabled index (col)")) -> (element=w669:dbl[])  [unwired: 1 in]
                          n305 = Index Array(array=w651, index (row)=1 ("disabled index (col)")) -> (element=w668:dbl[])  [unwired: 1 in]
                          n306 = local write "Averaged dt"(w664) -> ()
                          n307 = Bundle("B array"=w661, "Averaged P(B) Out"=w662) -> (w660:T7)  [unwired: 1 in]
                          n308 = Bundle("B array"=w661, "Averaged P(B) Out"=w663) -> (w659:T7)  [unwired: 1 in]
                          n309 = local write "Averaged P(B)"(w653) -> ()
                          n310 = Bundle("B array"=w661, "BaselineSubtracted I(B)"=w669) -> (w674:T8)  [unwired: 1 in]
                          n311 = Bundle("B array"=w661, "BaselineSubtracted I(B)"=w668) -> (w673:T8)  [unwired: 1 in]
                          n312 = Build Array(w660, w659) -> (→"P(B) /Averaged/":T9)
                          n313 = Build Array(w674, w673) -> (→"I(B) /Averaged/":T10)
                        }
                        frame True {
                          n314 = local read "T array"() -> (w689:dbl[])
                          n315 = local read "Counter"() -> (w702:i8)
                          n316 = local read "Averaged I(T)"() -> (w681:dbl[][])
                          n317 = local read "Up/Down"() -> (w705:bool)
                          n318 = local read "Averaged dt"() -> (w680:dbl[][])
                          n319 = local read "Sample area (mm^2)"() -> (w685:dbl)
                          n320 = call "Average_ITP_curves.vi"("I in"=w703, "Averaged P(T) In"="Averaged P(T)", "Counter"=w702, "Averaged I(T) In"=w681, "t in"=w694, "T in"=w704, "Averaged dt in"=w680, "Up/Down"=w705, "Sample area(mm^2)"=w685, "T array"=w689) -> ("Averaged I(B) out"=w679:dbl[][], "Averaged dt Out"=w692:dbl[][], "Averaged P(T) Out"=w682:dbl[][])  [unwired: 3 in]
                          "Averaged I(T)" <- w679
                          n321 = Index Array(array=w682, index (row)=0 ("disabled index (col)")) -> (element=w690:dbl[])  [unwired: 1 in]
                          n322 = Index Array(array=w682, index (row)=1 ("disabled index (col)")) -> (element=w691:dbl[])  [unwired: 1 in]
                          n323 = Index Array(array=w679, index (row)=0 ("disabled index (col)")) -> (element=w696:dbl[])  [unwired: 1 in]
                          n324 = Index Array(array=w679, index (row)=1 ("disabled index (col)")) -> (element=w695:dbl[])  [unwired: 1 in]
                          n325 = local write "Averaged dt"(w692) -> ()
                          n326 = Bundle("T array"=w689, "Averaged P(T) Out"=w690) -> (w688:T11)  [unwired: 1 in]
                          n327 = Bundle("T array"=w689, "Averaged P(T) Out"=w691) -> (w687:T11)  [unwired: 1 in]
                          n328 = local write "Averaged P(T)"(w682) -> ()
                          n329 = Bundle("T array"=w689, "Averaged I(B) out"=w696) -> (w701:T12)  [unwired: 1 in]
                          n330 = Bundle("T array"=w689, "Averaged I(B) out"=w695) -> (w700:T12)  [unwired: 1 in]
                          n331 = Build Array(w688, w687) -> (→"P(T) /Averaged/":T13)
                          n332 = Build Array(w701, w700) -> (→"I(T) /Averaged/":T14)
                        }
                      }
                    }
                    frame #1 {
                      # "Save and Reset"
                      n333 = local read "Sweep"() -> (w706:bool)
                      n334 = local read "Measurement File"() -> (w708:path)
                      n335 = local read "P(uC/mm^2)"() -> (w714:dbl[])
                      n336 = Build Array(w717, w716, w715, w713, w714) -> (w707:dbl[][])
                      n337 = case shown="True" w706 {
                        tunnel: w707 -> [_ w724]
                        frame False {
                        }
                        frame True {
                          n338 = local read "Up/Down"() -> (w720:bool)
                          n339 = case shown="True" w720 {
                            tunnel: [w725 w726] -> w719
                            frame False {
                              n340 = local read "Measurement File_dn"() -> (w725:path)
                            }
                            frame True {
                              n341 = local read "Measurement File_up"() -> (w726:path)
                            }
                          }
                          n342 = call-poly <vilib>:"Write Delimited Spreadsheet.vi"("file path (dialog if empty)"=w719, "format (%.3f)"="%.5g", "2D data"=w724, "append to file? (F)"=TRUE ("transpose? (F)"), "transpose? (F)"=FALSE ("append to file? (F)")) -> ()  [unwired: 9 in, 2 out]
                        }
                      }
                      n343 = case shown="False" "Reset IB?" {
                        frame False {
                        }
                        frame True {
                          n344 = local read "Up/Down"() -> (w727:bool)
                          n345 = case shown="False" w727 {
                            frame False {
                              n346 = invoke on="I(B) 3" class="XYGraph (strict)" method="Reinit To Default"() -> ()  [unwired: 3 in, 3 out]
                              n347 = invoke on="I(T)" class="XYGraph (strict)" method="Reinit To Default"() -> ()  [unwired: 3 in, 3 out]
                            }
                            frame True {
                            }
                          }
                        }
                      }
                      n348 = call-poly <vilib>:"Write Delimited Spreadsheet.vi"("file path (dialog if empty)"=w708, "format (%.3f)"="%.5g", "2D data"=w707, "append to file? (F)"=TRUE, "transpose? (F)"=TRUE) -> ()  [unwired: 9 in, 2 out]
                      n349 = local write "Reset"(FALSE ("Save")) -> ()
                    }
                    frame #2 {
                      w728 = dbl[] []
                      n350 = local write "P(uC/mm^2)"(w728) -> ()
                    }
                  }
                }
              }
              n351 = local read "New"() -> (w621:bool)
              n352 = case shown="False" w621 {
                tunnel: [Mode."Return" ("Enum") Mode."New" ("Enum")] -> w633
                tunnel: [TRUE FALSE] -> w620
                frame False {
                }
                frame True {
                }
              }
            }
            frame "New" {
              n353 = stacked-sequence {
                seq-local: [_ _ _ _ w844 _ _] -> [_ _ _ _ _ w871 _]
                seq-local: [_ _ w788 _ _ _ _] -> [_ _ _ _ w850 _ _]
                tunnel: T6 {"Com Port"=1, "ISOBUS Address"=0, "GPIB Address"=25, "Communication"=enum."GPIB"} ("Address") -> [_ _ w787 w832 _ _ _]
                tunnel: w731 -> [_ _ w789 _ _ w872 _]
                tunnel: [_ _ _ _ _ w874 _] -> w730
                tunnel: w729 -> [_ w764 _ _ _ _ _]
                frame #0 {
                  w757 = 1 ("index (row)")
                  w756 = 0 ("index (row)")
                  # "Save averages"
                  n354 = local read "Measurement File_average"() -> (w744:path)
                  n355 = local read "Averaged P(B)"() -> (w755:dbl[][])
                  n356 = local read "Averaged dt"() -> (w753:dbl[][])
                  n357 = local read "I(B) /Averaged/"() -> (w745:cluster{"B array":dbl[], dbl[]}[])
                  n358 = Index Array(array=w753, index (row)=w756) -> (element=w754:dbl[])  [unwired: 1 in]
                  n359 = Index Array(array=w753, index (row)=w757) -> (element=w761:dbl[])  [unwired: 1 in]
                  n360 = Index Array(array=w745, index=1) -> (element=w749:cluster{"B array":dbl[], dbl[]})
                  n361 = Index Array(array=w745, index=0) -> (element=w748:cluster{"B array":dbl[], dbl[]})
                  n362 = Unbundle(w749) -> ("B array"=w759:dbl[], w760:dbl[])
                  n363 = Unbundle(w748) -> ("B array"=w750:dbl[], w751:dbl[])
                  n364 = Index Array(array=w755, index (row)=w756) -> (element=w758:dbl[])  [unwired: 1 in]
                  n365 = Index Array(array=w755, index (row)=w757) -> (element=w762:dbl[])  [unwired: 1 in]
                  n366 = Build Array(w750, w751, w754, w758, w759, w760, w761, w762) -> (w752:dbl[][])
                  n367 = call-poly <vilib>:"Write Delimited Spreadsheet.vi"("file path (dialog if empty)"=w744, "format (%.3f)"="%.5g", "2D data"=w752, "append to file? (F)"=TRUE ("transpose? (F)"), "transpose? (F)"=TRUE ("append to file? (F)")) -> ()  [unwired: 9 in, 2 out]
                }
                frame #1 {
                  w770 = dbl[] []
                  w779 = dbl[] []
                  # "Reset Flags"
                  n368 = Get Date/Time In Seconds() -> (seconds since 1Jan1904=w780:timestamp)
                  n369 = local write "Up/Down"(TRUE ("Up/Down")) -> ()
                  n370 = local write "First?"(TRUE ("First?")) -> ()
                  n371 = local write "Offset?"(FALSE ("Offset?")) -> ()
                  n372 = local write "New"(FALSE ("New")) -> ()
                  n373 = local write "P(uC/mm^2)"(w779) -> ()
                  n374 = local write "Start time"(w780) -> ()
                  n375 = local write "Actual Polarization"(0.0 ("Actual Polarization")) -> ()
                  n376 = local write "Offset array"(w779) -> ()
                  n377 = local write "Up/Down"(TRUE ("Up/Down")) -> ()
                  n378 = local write "Reset"(FALSE ("Reset")) -> ()
                  n379 = local read "B array"() -> (w773:dbl[])
                  n380 = local write "Counter"(i8 0 ("Counter")) -> ()
                  n381 = invoke on="P(B)" class="XYGraph (strict)" method="Reinit To Default"() -> ()  [unwired: 3 in, 3 out]
                  n382 = invoke on="I(B) 3" class="XYGraph (strict)" method="Reinit To Default"() -> ()  [unwired: 3 in, 3 out]
                  n383 = Multiply(x=w773, y=0.0) -> (x*y=w774:dbl[])
                  n384 = Build Array(w770, w770) -> (w778:dbl[][])
                  n385 = Bundle("B array"=w773, w774) -> (w775:cluster{"B array":dbl[], dbl[]})  [unwired: 1 in]
                  n386 = local write "Averaged I(B)"(w778) -> ()
                  n387 = Build Array(w775, w775) -> (w776:cluster{"B array":dbl[], dbl[]}[])
                  n388 = local write "I(B) /Averaged/"(w776) -> ()
                  n389 = local write "Measuring"(FALSE ("Measuring")) -> ()
                  n390 = Flush Queue(queue=w764) -> (remaining elements=→"remaining elements 2":T1)  [unwired: 1 in, 2 out]
                }
                frame #2 {
                  # "Step"
                  n391 = local read "Sweep Rate Array"() -> (w793:dbl[])
                  n392 = local read "Channel B/A"() -> (w784:bool)
                  n393 = local read "j"() -> (w794:i32)
                  n394 = Increment(x=w794) -> (x+1=w790:i32)
                  n395 = Array Size(array=w793) -> (size(s)=w792:i32)
                  n396 = Less?(x=w790, y=w792) -> (x < y?=w791:bool)
                  "Step Rate" <- w791
                  n397 = Select(t="1,0  " ("write buffer"), s=w784, f="2,0  " ("write buffer")) -> (s? t:f=w783:string)
                  n398 = case shown="False" w791 {
                    tunnel: w790 -> [_ w825]
                    tunnel: w789 -> [w798 w824]
                    tunnel: [w797 w824] -> w788
                    tunnel: w787 -> [w796 _]
                    tunnel: w783 -> [w795 _]
                    frame False {
                      # "Step Temp?"
                      n399 = local read "Temperature Array"() -> (w802:dbl[])
                      n400 = local read "i"() -> (w803:i32)
                      n401 = Increment(x=w803) -> (x+1=w800:i32)
                      n402 = local write "j"(0 ("f")) -> ()
                      n403 = Array Size(array=w802) -> (size(s)=w801:i32)
                      n404 = Less?(x=w800, y=w801) -> (x < y?=w799:bool)
                      "Step Temp" <- w799
                      n405 = case shown="False" w799 {
                        tunnel: w800 -> [_ w823]
                        tunnel: w798 -> [w809 w822]
                        tunnel: [w808 w822] -> w797
                        tunnel: w796 -> [w807 _]
                        tunnel: w795 -> [w805 _]
                        frame False {
                          # "Heater OFF"
                          # "Finished"
                          n406 = local write "i"(0 ("i")) -> ()
                          n407 = stacked-sequence {
                            tunnel: w809 -> [w816 _ _]
                            tunnel: [w815 _ _] -> w808
                            tunnel: w807 -> [_ w819 w820]
                            tunnel: w805 -> [w813 _ _]
                            frame #0 {
                              n408 = Concatenate Strings("RANGE," ("write buffer"), w813) -> (w812:string)
                              n409 = local read "Lake Shore"() -> (w817:refnum<visa-resource-name>)
                              n410 = VISA Write(VISA resource name=w817, write buffer=w812, error in (no error)=w816) -> (error out=w815:errorcluster)  [unwired: 2 out]
                            }
                            frame #1 {
                              n411 = call "ips_switchHeaterOff.vi"("Instrument address"=w819, "Rate"=2.0) -> ()  [unwired: 1 out]
                            }
                            frame #2 {
                              n412 = call "GPIB - BusCommand.vi"("Command"="H0", "Address"=w820) -> ()  [unwired: 2 out]
                            }
                          }
                          n413 = local write "Record ALL"(FALSE ("Record ALL")) -> ()
                          "Finished" <- TRUE
                        }
                        frame True {
                          n414 = local write "i"(w823) -> ()
                        }
                      }
                    }
                    frame True {
                      n415 = local write "j"(w825) -> ()
                    }
                  }
                }
                frame #3 {
                  # "Set rates"
                  n416 = local read "Sweep Rate Array"() -> (w831:dbl[])
                  n417 = local read "j"() -> (w830:i32)
                  n418 = local read "j"() -> (w828:i32)
                  n419 = Index Array(array=w831, index=w830) -> (element=w829:dbl)
                  n420 = Number To Fractional String(number=w829, precision (6)=i16 3) -> (F-format string=w835:string)  [unwired: 2 in]
                  n421 = Index Array(array="Max count array", index=w828) -> (element=w826:i32)
                  n422 = local write "Max Countl"(w826) -> ()
                  n423 = Concatenate Strings("T" ("format string"), w835) -> (w836:string)
                  n424 = call "GPIB - BusCommand.vi"("Command"=w836, "Address"=w832) -> ()  [unwired: 2 out]
                  n425 = local write "Sweep Rate (T/min)"(w829) -> ()
                }
                frame #4 {
                  # "Set temperature"
                  n426 = local read "Temperature Array"() -> (w852:dbl[])
                  n427 = local read "i"() -> (w851:i32)
                  n428 = Index Array(array=w852, index=w851) -> (element=w849:dbl)
                  n429 = local read "Lake Shore"() -> (w853:refnum<visa-resource-name>)
                  n430 = local read "Channel B/A"() -> (w840:bool)
                  n431 = Number To Fractional String(number=w849, precision (6)=i16 3) -> (F-format string=w839:string)  [unwired: 2 in]
                  n432 = Select(t="1,  " ("write buffer"), s=w840, f="2,  " ("write buffer")) -> (s? t:f=w837:string)
                  n433 = Concatenate Strings("SETP " ("write buffer"), w837, w839) -> (w838:string)
                  n434 = VISA Write(VISA resource name=w853, write buffer=w838, error in (no error)=w850) -> (VISA resource name out=w846:refnum<visa-resource-name>, error out=w845:errorcluster)  [unwired: 1 out]
                  n435 = Greater?(x=w849, y=9.0) -> (0:w847:bool)
                  n436 = case shown="True" w847 {
                    tunnel: w846 -> [w859 w867]
                    tunnel: w845 -> [w858 w866]
                    tunnel: [w857 w865] -> w844
                    tunnel: w837 -> [w855 w863]
                    frame True {
                      n437 = Number To Decimal String(number=enum16{"Off", "Low", "Medium", "High"}."High" ("Heater Range 2")) -> (decimal integer string=w862:string)  [unwired: 1 in]
                      n438 = Concatenate Strings("RANGE," ("write buffer"), w855, w862) -> (w861:string)
                      n439 = VISA Write(VISA resource name=w859, write buffer=w861, error in (no error)=w858) -> (error out=w857:errorcluster)  [unwired: 2 out]
                    }
                    frame False {
                      n440 = Number To Decimal String(number=enum16{"Off", "Low", "Medium", "High"}."High" ("Heater Range 2")) -> (decimal integer string=w870:string)  [unwired: 1 in]
                      n441 = Concatenate Strings("RANGE," ("write buffer"), w863, w870) -> (w869:string)
                      n442 = VISA Write(VISA resource name=w867, write buffer=w869, error in (no error)=w866) -> (error out=w865:errorcluster)  [unwired: 2 out]
                    }
                  }
                }
                frame #5 {
                  n443 = local read "Finished"() -> (w873:bool)
                  n444 = case shown="False" w873 {
                    tunnel: [w888 w937] -> w874
                    tunnel: w872 -> [_ _]
                    tunnel: w871 -> [w885 w937]
                    frame False {
                      w883 = "_" ("string")
                      # "Wait, create Files"
                      n445 = local read "Temperature Array"() -> (w915:dbl[])
                      n446 = local read "Sweep Rate Array"() -> (w911:dbl[])
                      n447 = local read "i"() -> (w914:i32)
                      n448 = local read "j"() -> (w912:i32)
                      n449 = Index Array(array=w915, index=w914) -> (element=w913:dbl)
                      n450 = Index Array(array=w911, index=w912) -> (element=w880:dbl)
                      n451 = Round Toward -Infinity(1:w880) -> (0:w881:dbl)
                      n452 = Number To Fractional String(use system decimal point (T)=TRUE, number=w913, precision (6)=i16 1) -> (F-format string=w875:string)  [unwired: 1 in]
                      n453 = Subtract(x=w880, y=w881) -> (x-y=w882:dbl)
                      n454 = Equal To 0?(x=w882) -> (x = 0?=w879:bool)
                      n455 = Select(t=i16 0 ("precision (6)"), s=w879, f=i16 2 ("precision (6)")) -> (s? t:f=w876:i16)
                      n456 = Number To Fractional String(use system decimal point (T)=TRUE, number=w880, precision (6)=w876) -> (F-format string=w884:string)  [unwired: 1 in]
                      n457 = Concatenate Strings("Directory", "\\" ("string"), "FileName", w883, w875, "K" ("string"), w883, w884, "Tpm" ("string")) -> (w905:string)
                      n458 = local read "Step Temp"() -> (w889:bool)
                      n459 = local write "Step Rate"(FALSE ("Step Rate")) -> ()
                      n460 = Search and Replace String(replace all?=TRUE ("replace all? (F)"), input string=w905, search string=".", replace string="p" ("substring (\"\")"), error in=w885) -> (result string=w900:string, error out=w895:errorcluster)  [unwired: 3 in, 2 out]
                      n461 = Concatenate Strings(w900, ".txt" ("string")) -> (w899:string)
                      n462 = case shown="True" w889 {
                        tunnel: w875 -> [_ w917]
                        frame False {
                        }
                        frame True {
                          n463 = stacked-sequence {
                            tunnel: w917 -> [_ w929 _]
                            frame #0 {
                              n464 = Get Date/Time In Seconds() -> (seconds since 1Jan1904=w918:timestamp)
                              n465 = while {
                                tunnel: w918 -> [w922]
                                stop <- w919 stop-if-true
                                n466 = Get Date/Time In Seconds() -> (seconds since 1Jan1904=w923:timestamp)
                                n467 = Subtract(x=w923, y=w922) -> (x-y=w921:dbl)
                                "Wait (s)" <- w921
                                n468 = Greater Or Equal?(x=w921, y="secs to wait") -> (x >= y?=w919:bool)
                              }
                            }
                            frame #1 {
                              n469 = local read "Directory"() -> (w925:string)
                              n470 = Concatenate Strings(w925, "\\" ("string"), w929, "K_calib" ("string"), ".txt" ("string")) -> (w930:string)
                              n471 = String To Path(string=w930) -> (path=w927:path)
                              n472 = call "Calibration_Hall_full.vi"() -> ("Calibration Curve"=w934:cluster{dbl[], "Best Linear Fit":dbl[]}[], "Calibration Curve Data"=w931:dbl[][])  [unwired: 10 in]
                              n473 = local write "Step Temp"(FALSE ("Step Temp")) -> ()
                              n474 = Transpose 2D Array(2D array=w931) -> (transposed array=w932:dbl[][])
                              n475 = local write "Calibration Curve Data"(w931) -> ()
                              n476 = call-poly <vilib>:"Write Delimited Spreadsheet.vi"("file path (dialog if empty)"=w927, "format (%.3f)"="%.8f", "2D data"=w932) -> ()  [unwired: 11 in, 2 out]
                              n477 = local write "Calibration Curve"(w934) -> ()
                            }
                            frame #2 {
                              n478 = Wait (ms)(milliseconds to wait=u32 60000) -> ()  [unwired: 1 out]
                            }
                          }
                        }
                      }
                      n479 = String To Path(string=w899) -> (path=w898:path)
                      n480 = Open/Create/Replace File(file path (use dialog)=w898, error in=w895, operation (0:open)=T5."open or create") -> (refnum out=w887:refnum<file>, error out=w888:errorcluster)  [unwired: 3 in, 1 out]
                      n481 = local write "refnum out"(w887) -> ()
                      n482 = Refnum to Path(1:w887) -> (0:w890:path)
                      n483 = call "Create_sweep_files.vi"("Measurement File"=w890) -> ("Path 3"=w893:path, "Path 2"=w892:path, "Path"=w891:path)  [unwired: 8 in]
                      n484 = local write "Measurement File"(w890) -> ()
                      n485 = local write "Measurement File_dn"(w893) -> ()
                      n486 = local write "Measurement File_average"(w891) -> ()
                      n487 = local write "Measurement File_up"(w892) -> ()
                    }
                    frame True {
                    }
                  }
                }
                frame #6 {
                  n488 = local read "Finished"() -> (w938:bool)
                  n489 = case shown="True" w938 {
                    frame False {
                      n490 = local write "Measuring"(TRUE ("Measuring")) -> ()
                    }
                    frame True {
                      n491 = local write "Measure /Pause"(FALSE ("Measure /Pause")) -> ()
                    }
                  }
                }
              }
            }
            frame "Return" {
            }
          }
        }
      }
      frame Error {
        # "Return true for any case which should stop the loop."
      }
    }
  }
  n492 = VISA Read(VISA resource name=w10, byte count=u32 100, error in (no error)=w12) -> (VISA resource name out=w9:refnum<visa-resource-name>, read buffer=w8:string, error out=w11:errorcluster)  [unwired: 1 out]
  n493 = VISA Open(error in (no error)=w11, VISA resource name="Magnetic Field") -> (VISA resource name=w105:refnum<visa-resource-name>, error out=w87:errorcluster)  [unwired: 3 in]
  n494 = VISA Open(error in (no error)=w87, VISA resource name="Lake Shore") -> (VISA resource name=w82:refnum<visa-resource-name>, error out=w51:errorcluster)  [unwired: 3 in]
  n495 = VISA Write(VISA resource name="Lake Shore", write buffer="KRDG?b", error in (no error)=w51) -> (VISA resource name out=w48:refnum<visa-resource-name>, error out=w47:errorcluster)  [unwired: 1 out]
  n496 = VISA Read(VISA resource name=w48, byte count=w54, error in (no error)=w47) -> (VISA resource name out=w45:refnum<visa-resource-name>, read buffer=w59:string, error out=w46:errorcluster)  [unwired: 1 out]
  n497 = VISA Write(VISA resource name=w45, write buffer="SETP?b", error in (no error)=w46) -> (VISA resource name out=w44:refnum<visa-resource-name>, error out=w43:errorcluster)  [unwired: 1 out]
  n498 = VISA Read(VISA resource name=w44, byte count=w54, error in (no error)=w43) -> (VISA resource name out=w41:refnum<visa-resource-name>, read buffer=w58:string, error out=w42:errorcluster)  [unwired: 1 out]
  n499 = VISA Write(VISA resource name=w41, write buffer="RANGE?b", error in (no error)=w42) -> (VISA resource name out=w39:refnum<visa-resource-name>, error out=w40:errorcluster)  [unwired: 1 out]
  n500 = Fract/Exp String To Number(string=w59) -> (number=w57:dbl)  [unwired: 3 in, 1 out]
  n501 = VISA Read(VISA resource name=w39, byte count=w54, error in (no error)=w40) -> (read buffer=w53:string, error out=w50:errorcluster)  [unwired: 2 out]
  n502 = Fract/Exp String To Number(string=w58) -> (number=w56:dbl)  [unwired: 3 in, 1 out]
  n503 = Fract/Exp String To Number(string=w53) -> (number=w49:dbl)  [unwired: 3 in, 1 out]
  n504 = local write "Actual Temperature (K)"(w57) -> ()
  n505 = local write "Setpoint Temperature (K)"(w56) -> ()
  n506 = local write "Heater Range"(w49) -> ()
  n507 = case shown="True" w64 {
    frame False {
    }
    frame True {
      n508 = invoke on="P(T)" class="XYGraph (strict)" method="Reinit To Default"() -> ()  [unwired: 3 in, 3 out]
      n509 = invoke on="I(T)" class="XYGraph (strict)" method="Reinit To Default"() -> ()  [unwired: 3 in, 3 out]
    }
  }
  n510 = Decimal String To Number(string=w8) -> (number=w7:i32)  [unwired: 2 in, 1 out]
  n511 = local write "Keithley (IV conv) averaging"(w7) -> ()
  n512 = while {
    shift-right: [w969] -> w103
    shift-left: w84 -> [w970]
    shift-right: [w971] -> w108
    shift-left: w109 -> [w972]
    tunnel: w9 -> [w968]
    tunnel: w105 -> [w967]
    tunnel: w50 -> [_]
    tunnel: [w961] -> _
    tunnel: w92 -> [w960]
    tunnel: w82 -> [w959]
    tunnel: w17 -> [w958]
    stop <- "stop" stop-if-true
    n513 = event shown="[10] \"Calibrate\": Value Change" {
      selector: _ -> [_ _ _ _ _ _ _ _ _ _ _ _ _ _ _ _]
      dyn-events: _ -> [_ _ _ _ _ _ _ _ _ _ _ _ _ _ _ _]
      timeout: 10 -> [_ _ _ _ _ _ _ _ _ _ _ _ _ _ _ _]
      tunnel: w972 -> [w982 w1028 w1046 w1056 w1070 w1126 w1130 w1134 w1172 w1188 w1205 w1235 w1252 w1273 w1288 w1297]
      tunnel: [w981 w1028 w1046 w1056 w1070 w1126 w1130 w1134 w1172 w1188 w1205 w1235 w1252 w1273 w1288 w1297] -> w971
      tunnel: w970 -> [w980 w1037 w1045 w1055 w1068 w1125 w1132 w1136 w1173 w1187 w1204 w1236 w1254 w1277 w1292 w1299]
      tunnel: [w979 w1029 w1045 w1055 w1067 w1127 w1132 w1135 _ w1187 w1204 w1236 w1253 w1276 w1291 w1298] -> w969
      tunnel: w968 -> [w978 w1038 _ _ _ _ _ _ _ _ _ _ _ _ _ _]
      tunnel: w967 -> [w977 _ _ _ _ _ _ _ _ _ _ _ _ _ _ _]
      tunnel: [w975 w1027 w1044 w1054 w1069 w1128 w1131 w1133 w1171 w1186 w1203 w1234 w1251 w1274 w1289 _] -> w961
      tunnel: w960 -> [w975 w1027 w1044 w1057 w1069 w1128 w1131 w1133 w1171 w1186 w1203 w1234 w1251 w1274 w1289 _]
      tunnel: w959 -> [_ _ _ _ _ _ _ _ _ _ _ _ w1255 w1275 w1293 w1296]
      tunnel: [_ _ _ _ _ _ _ _ w1173 _ _ _ _ _ _ _] -> _
      tunnel: w958 -> [w974 _ _ _ _ _ _ _ _ _ _ _ _ _ _ _]
      event Timeout {
        n514 = event-data() -> ()  [unwired: 1 in, 3 out]
        n515 = case shown="True" "Measuring" {
          tunnel: w982 -> [w984 w1007]
          tunnel: [w984 w1006] -> w981
          tunnel: w980 -> [w983 w985]
          tunnel: [w983 w1005] -> w979
          tunnel: w978 -> [_ w998]
          tunnel: w977 -> [_ w997]
          tunnel: w974 -> [_ w988]
          frame False {
          }
          frame True {
            w996 = ":FETCh? " ("data")
            w999 = u32 1000 ("byte count")
            # "Generate the data here."
            n516 = case shown="No Error" w985 {
              selector: w985 -> [w1019 w1020]
              tunnel: [w1019 w1020] -> w993
              tunnel: [w1018 _] -> w992
              frame No Error {
                n517 = Get Date/Time In Seconds() -> (seconds since 1Jan1904=w1018:timestamp)
              }
              frame Error {
              }
            }
            n518 = VISA Write(VISA resource name=w998, write buffer=w996, error in (no error)=w993) -> (VISA resource name out=w1004:refnum<visa-resource-name>, error out=w1002:errorcluster)  [unwired: 1 out]
            n519 = VISA Write(VISA resource name=w997, write buffer=w996, error in (no error)=w1002) -> (VISA resource name out=w1003:refnum<visa-resource-name>, error out=w1001:errorcluster)  [unwired: 1 out]
            n520 = VISA Read(VISA resource name=w1004, byte count=w999, error in (no error)=w1001) -> (read buffer=w994:string, error out=w1000:errorcluster)  [unwired: 2 out]
            n521 = VISA Read(VISA resource name=w1003, byte count=w999, error in (no error)=w1000) -> (read buffer=w995:string, error out=w990:errorcluster)  [unwired: 2 out]
            n522 = case shown="False" "DaQ" {
              tunnel: w990 -> [w1009 w1015]
              tunnel: [w1009 w1014] -> w989
              tunnel: w988 -> [_ w1013]
              tunnel: [0.0 ("Output") w1011] -> w986
              frame False {
              }
              frame True {
                n523 = local read "Number of Samples"() -> (w1017:i32)
                n524 = call-poly <vilib>:"DAQmx Read.vi"("task/channels in"=w1013, "number of samples per channel"=w1017, "error in"=w1015) -> ("data"=w1016:dbl[], "error out"=w1014:errorcluster)  [unwired: 10 in, 1 out]
                n525 = call-poly <vilib>:"Mean.vi"("X"=w1016) -> ("mean"=w1012:dbl)  [unwired: 1 out]
                "Actual mean" <- w1012
                n526 = call "N Point Running Average.vi"("n"="Moving average", "Input"=w1012) -> ("Output"=w1011:dbl)
              }
            }
            n527 = Bundle("seconds since 1Jan1904"=w992, "read buffer"=w994, "read buffer"=w995, "Output"=w986) -> (w991:T4)  [unwired: 1 in]
            n528 = Enqueue Element(queue=w1007, element=w991, error in (no error)=w989) -> (queue out=w1006:refnum<queue>, error out=w1005:errorcluster)  [unwired: 1 in, 1 out]
          }
        }
      }
      event "Keithley (IV conv) averaging": Value Change {
        n529 = event-data() -> ()  [unwired: 1 in, 6 out]
        n530 = Number To Decimal String(number="Keithley (IV conv) averaging") -> (decimal integer string=w1035:string)  [unwired: 1 in]
        n531 = Concatenate Strings("VOLTage:DC:AVERage:COUNt " ("write buffer"), w1035) -> (w1034:string)
        n532 = VISA Write(VISA resource name=w1038, write buffer=w1034, error in (no error)=w1037) -> (VISA resource name out=w1033:refnum<visa-resource-name>, error out=w1031:errorcluster)  [unwired: 1 out]
        n533 = VISA Write(VISA resource name=w1033, write buffer="VOLTage:DC:AVERage:COUNt?", error in (no error)=w1031) -> (VISA resource name out=w1026:refnum<visa-resource-name>, error out=w1030:errorcluster)  [unwired: 1 out]
        n534 = VISA Read(VISA resource name=w1026, byte count=u32 100, error in (no error)=w1030) -> (read buffer=w1024:string, error out=w1029:errorcluster)  [unwired: 2 out]
        n535 = Decimal String To Number(string=w1024) -> (number=w1023:i32)  [unwired: 2 in, 1 out]
        n536 = Equal?(x="Keithley (IV conv) averaging", y=w1023) -> (x = y?=→"Confirm":bool)
      }
      event "Max Field (T)": Value Change {
        n537 = event-data() -> ()  [unwired: 1 in, 6 out]
        n538 = Divide(x="Max Field (T)", y="dB (T)") -> (x/y=w1041:dbl)
        n539 = for {
          N: w1041 -> [_]
          tunnel: "dB (T)" -> [w1051]
          tunnel: [w1048] -> w1040 mode=indexing
          tunnel: "Min Field (T)" -> [w1049]
          tunnel: [0.0] -> _ mode=indexing
          i -> [w1052]
          n540 = Multiply(x=w1052, y=w1051) -> (x*y=w1050:dbl)
          n541 = Add(x=w1050, y=w1049) -> (x+y=w1048:dbl)
        }
        "B array" <- w1040
      }
      event "Sweep Rate (T/min)": Value Change {
        n542 = event-data() -> ("NewVal"=w1058:dbl)  [unwired: 1 in, 5 out]
        n543 = local read "Magnet"() -> (w1053:bool)
        n544 = case shown="False" w1053 {
          tunnel: w1058 -> [_ w1065]
          tunnel: w1057 -> [w1059 w1061]
          tunnel: [w1059 w1060] -> w1054
          frame False {
          }
          frame True {
            n545 = Number To Fractional String(number=w1065, precision (6)=i16 3) -> (F-format string=w1063:string)  [unwired: 2 in]
            n546 = Concatenate Strings("T" ("format string"), w1063) -> (w1062:string)
            n547 = call "GPIB - BusCommand.vi"("Command"=w1062, "Address"=w1061) -> ("Address(thru)"=w1060:T6)  [unwired: 1 out]
          }
        }
      }
      event "Field To Zero": Value Change {
        n548 = event-data() -> ()  [unwired: 1 in, 6 out]
        n549 = Two Button Dialog(message="Do you want to switch off the field?", 1:"No" ("F button name (\"Cancel\")"), 2:"Yes" ("T button name (\"OK\")")) -> (T button?=w1074:bool)
        n550 = case shown="True" w1074 {
          tunnel: w1069 -> [_ w1079]
          tunnel: w1068 -> [w1075 w1077]
          tunnel: [w1075 w1076] -> w1067
          frame False {
          }
          frame True {
            n551 = local read "Magnet"() -> (w1078:bool)
            n552 = case shown="False" w1078 {
              tunnel: w1079 -> [_ w1118]
              tunnel: w1077 -> [w1082 w1115]
              tunnel: [w1081 w1115] -> w1076
              frame False {
                n553 = local read "Lock_in_Amplifier"() -> (w1080:refnum<visa-resource-name>)
                n554 = stacked-sequence {
                  seq-local: [w1085 _] -> [_ w1098]
                  seq-local: [w1083 _] -> [_ w1095]
                  tunnel: w1082 -> [w1087 _]
                  tunnel: [_ w1099] -> w1081
                  tunnel: w1080 -> [w1084 w1096]
                  frame #0 {
                    n555 = VISA Write(VISA resource name=w1084, write buffer="AUXV?1", error in (no error)=w1087) -> (VISA resource name out=w1091:refnum<visa-resource-name>, error out=w1086:errorcluster)  [unwired: 1 out]
                    n556 = VISA Read(VISA resource name=w1091, byte count=u32 1000, error in (no error)=w1086) -> (read buffer=w1088:string, error out=w1085:errorcluster)  [unwired: 2 out]
                    n557 = Fract/Exp String To Number(string=w1088) -> (number=w1083:dbl)  [unwired: 3 in, 1 out]
                  }
                  frame #1 {
                    w1102 = 0.001 ("Voltage Step (V)")
                    n558 = local read "Sweep Rate (T/min)"() -> (w1101:dbl)
                    n559 = xnode "Sweep Delay"("SweepRate"=w1101, "Resolution"=w1102) -> ("Result"=w1100:dbl)  [unwired: 2 in, 1 out]
                    n560 = call "Universal_Ramping.vi"("milliseconds to wait"=w1100, "Initial Voltage (V)"=w1095, "error in (no error)"=w1098, "Voltage Step (V)"=w1102, "Final Voltage (V)"=0.0, "VISA resource name"=w1096) -> ("error out"=w1099:errorcluster, "Actual Voltage (V)"=w1092:dbl)  [unwired: 3 in, 1 out]
                    n561 = local read "Calibration Curve Data"() -> (w1094:dbl[][])
                    n562 = local write "Hall Resistance (Ohm)"(w1092) -> ()
                    n563 = call "HallR_to_B.vi"("Measured R(Ohm)"=w1092, "Calibration Curve Data"=w1094) -> ("Interpolated B value"=w1093:dbl)  [unwired: 9 in]
                    n564 = local write "Actual B Field (T)"(w1093) -> ()
                  }
                }
              }
              frame True {
                n565 = local read "Sweep Rate (T/min)"() -> (w1117:dbl)
                n566 = call "ips_switchHeaterOff.vi"("Instrument address"=w1118, "Rate"=w1117) -> ("B"=w1116:dbl)
                n567 = local write "Nominal Field (T)"(w1116) -> ()
              }
            }
          }
        }
      }
      event "Go to Set": Value Change {
        n568 = event-data() -> ()  [unwired: 1 in, 6 out]
        n569 = local read "Lock_in_Amplifier"() -> (w1121:refnum<visa-resource-name>)
        n570 = local read "Sweep Rate (T/min)"() -> (w1123:dbl)
        n571 = local read "Magnet"() -> (w1124:bool)
        n572 = call "Ramp_Field.vi"("Set Field (T) in"="Set Field (T)", "Sweep Rate (T/min)"=w1123, "error in (no error)"=w1125, "Magnet"=w1124, "VISA Refnum in"=w1121) -> ("error out"=w1127:errorcluster, "Actual Voltage (V)"=w1119:dbl, "Set Field (T) out"=w1122:dbl)  [unwired: 4 in]
        n573 = local write "Actual B Field (T)"(w1122) -> ()
        n574 = local write "Hall Resistance (Ohm)"(w1119) -> ()
      }
      event "Measure /Pause": Value Change {
        n575 = event-data() -> ("NewVal"=w1129:bool)  [unwired: 1 in, 5 out]
        n576 = local write "Measuring"(w1129) -> ()
      }
      event "Stop": Value Change {
        n577 = event-data() -> ()  [unwired: 1 in, 6 out]
        n578 = local read "Measuring"() -> (w1137:bool)
        n579 = case shown="True" w1137 {
          tunnel: w1136 -> [w1138 w1141]
          tunnel: [w1138 w1142] -> w1135
          frame False {
          }
          frame True {
            w1147 = FALSE ("Measuring")
            n580 = local read "SaveSweep"() -> (w1148:bool)
            n581 = local write "Measuring"(w1147) -> ()
            n582 = local write "Measure /Pause"(w1147) -> ()
            n583 = local read "Lock_in_Amplifier"() -> (w1143:refnum<visa-resource-name>)
            n584 = case shown="True" w1148 {
              frame False {
              }
              frame True {
                w1154 = 1 ("index (row)")
                w1155 = 0 ("index (row)")
                n585 = local read "Measurement File_average"() -> (w1167:path)
                n586 = local read "Averaged P(B)"() -> (w1156:dbl[][])
                n587 = local read "Averaged dt"() -> (w1158:dbl[][])
                n588 = local read "I(B) /Averaged/"() -> (w1166:cluster{"B array":dbl[], dbl[]}[])
                n589 = Index Array(array=w1158, index (row)=w1155) -> (element=w1157:dbl[])  [unwired: 1 in]
                n590 = Index Array(array=w1158, index (row)=w1154) -> (element=w1150:dbl[])  [unwired: 1 in]
                n591 = Index Array(array=w1166, index=1) -> (element=w1162:cluster{"B array":dbl[], dbl[]})
                n592 = Index Array(array=w1166, index=0) -> (element=w1163:cluster{"B array":dbl[], dbl[]})
                n593 = Unbundle(w1162) -> ("B array"=w1152:dbl[], w1151:dbl[])
                n594 = Unbundle(w1163) -> ("B array"=w1161:dbl[], w1160:dbl[])
                n595 = Index Array(array=w1156, index (row)=w1155) -> (element=w1153:dbl[])  [unwired: 1 in]
                n596 = Index Array(array=w1156, index (row)=w1154) -> (element=w1149:dbl[])  [unwired: 1 in]
                n597 = Build Array(w1161, w1160, w1157, w1153, w1152, w1151, w1150, w1149) -> (w1159:dbl[][])
                n598 = call-poly <vilib>:"Write Delimited Spreadsheet.vi"("file path (dialog if empty)"=w1167, "format (%.3f)"="%.5g", "2D data"=w1159, "append to file? (F)"=TRUE ("transpose? (F)"), "transpose? (F)"=TRUE ("append to file? (F)")) -> ()  [unwired: 9 in, 2 out]
              }
            }
            n599 = local read "Sweep Rate (T/min)"() -> (w1145:dbl)
            n600 = local read "Set Field (T)"() -> (w1146:dbl)
            n601 = local read "Magnet"() -> (w1144:bool)
            n602 = call "Ramp_Field.vi"("Set Field (T) in"=w1146, "Sweep Rate (T/min)"=w1145, "error in (no error)"=w1141, "Magnet"=w1144, "VISA Refnum in"=w1143) -> ("error out"=w1142:errorcluster, "Actual Voltage (V)"=w1139:dbl, "Set Field (T) out"=w1140:dbl)  [unwired: 4 in]
            n603 = local write "Actual B Field (T)"(w1140) -> ()
            n604 = local write "Hall Resistance (Ohm)"(w1139) -> ()
          }
        }
      }
      event "Sweep": Value Change {
        n605 = event-data() -> ("NewVal"=w1174:bool)  [unwired: 1 in, 5 out]
        n606 = case shown="True" w1174 {
          frame False {
          }
          frame True {
            n607 = local read "Measurement File"() -> (w1175:path)
            n608 = Two Button Dialog(message="Do you want to create additional files for the sweeping measurements?" ("string"), 1:"No" ("F button name (\"Cancel\")"), 2:"Yes" ("T button name (\"OK\")")) -> (T button?=w1177:bool)
            n609 = case shown="True" w1177 {
              tunnel: w1175 -> [_ w1182]
              frame False {
                n610 = local write "SaveSweep"(FALSE ("SaveSweep")) -> ()
              }
              frame True {
                n611 = call "Create_sweep_files.vi"("Measurement File"=w1182) -> ("Path 3"=→"Measurement File_dn":path, "Path 2"=→"Measurement File_up":path, "Path"=→"Measurement File_average":path)  [unwired: 8 in]
                "SaveSweep" <- TRUE
              }
            }
          }
        }
      }
      event "Measure Noise": Value Change {
        n612 = event-data() -> ("NewVal"=w1189:bool)  [unwired: 1 in, 5 out]
        n613 = case shown="True" w1189 {
          frame False {
          }
          frame True {
            n614 = local read "Gain (V/A)"() -> (w1194:dbl)
            n615 = call "Noise_measurement.vi"("Gain (V/A)"=w1194, "Cycles"="Cycles", "Lower Cut-Off"="Cut-Off Frequency", "minimum value"="minimum value", "Filter On"="Filter On", "maximum value"="maximum value", "physical channels"="physical channels", "rate"="Rate", "samples per channel"="Samples per channel") -> ("Current (pA) Filtered"=→"Current (pA) Filtered":waveform(dbl), "PSD (pA/Hz^1/2) Peaks Removed"=→"PSD (pA/Hz^1/2) Peaks Removed":cluster{"f0":dbl, "df":dbl, "magnitude":dbl[]}, "Current (pA)"=→"Current (pA)":dbl[], "PSD (pA/Hz^1/2)"=→"PSD (pA/Hz^1/2)":cluster{"f0":dbl, "df":dbl, "magnitude":dbl[]})  [unwired: 3 in]
          }
        }
      }
      event "Calibrate": Value Change {
        n616 = event-data() -> ()  [unwired: 1 in, 6 out]
        n617 = case shown="True" "Calibrate" {
          frame False {
          }
          frame True {
            w1208 = dbl[] []
            n618 = while {
              shift-right: [w1225] -> _
              shift-left: w1208 -> [w1226]
              shift-right: [w1219] -> _
              shift-left: w1208 -> [w1220]
              shift-right: [w1222] -> _
              shift-left: "Start Field" -> [w1221]
              tunnel: [w1217] -> w1209
              stop <- w1227 stop-if-true
              n619 = call "Calibration_Hall.vi"("Dwell Time (ms)"="Dwell Time (ms)", "R array in (V)"=w1220, "Max Field"="Max Field", "B array in (T)"=w1226, "Set Field (T)"=w1221, "dB"="dB") -> ("R array out (V)"=w1219:dbl[], "Ready?"=w1229:bool, 14:"Calibration Curve"=w1217:dbl[][], 15:"Calibration Curve"=→"Calibration Curve":cluster{dbl[], dbl[]}[], "B array Out"=w1225:dbl[], "Set Field out"=w1222:dbl)  [unwired: 8 in]
              "Calibration Curve Data" <- w1217
              n620 = Or(x=w1229, y="stop 2") -> (x .or. y?=w1227:bool)
            }
            n621 = flat-sequence {
              tunnel: w1209 -> [w1212]
              frame #0 {
                n622 = Two Button Dialog(message="Do you want to save calibration file?") -> (T button?=w1211:bool)  [unwired: 2 in]
                n623 = case shown="True" w1211 {
                  tunnel: w1212 -> [_ w1215]
                  frame False {
                  }
                  frame True {
                    n624 = Transpose 2D Array(2D array=w1215) -> (transposed array=w1213:dbl[][])
                    n625 = call-poly <vilib>:"Write Delimited Spreadsheet.vi"("format (%.3f)"="%.8f", "2D data"=w1213) -> ()  [unwired: 12 in, 2 out]
                  }
                }
              }
            }
          }
        }
      }
      event "New Measurement File": Value Change {
        n626 = event-data() -> ()  [unwired: 1 in, 6 out]
        n627 = local read "Sweep"() -> (w1231:bool)
        n628 = Open/Create/Replace File(prompt="Please select measurement file\n", operation (0:open)=T5."replace or create with confirmation") -> (refnum out=w1237:refnum<file>)  [unwired: 4 in, 2 out]
        n629 = local write "refnum out"(w1237) -> ()
        n630 = Refnum to Path(1:w1237) -> (0:w1232:path)
        n631 = case shown="True" w1231 {
          tunnel: w1232 -> [_ w1240]
          frame False {
          }
          frame True {
            n632 = Two Button Dialog(message="Do you want to create additional files for the sweeping measurements?" ("string"), 1:"No" ("F button name (\"Cancel\")"), 2:"Yes" ("T button name (\"OK\")")) -> (T button?=w1242:bool)
            n633 = case shown="True" w1242 {
              tunnel: w1240 -> [_ w1250]
              frame False {
                n634 = local write "SaveSweep"(FALSE ("SaveSweep")) -> ()
              }
              frame True {
                n635 = call "Create_sweep_files.vi"("Measurement File"=w1250) -> ("Path 3"=w1247:path, "Path 2"=w1248:path, "Path"=w1249:path)  [unwired: 8 in]
                n636 = local write "Measurement File_dn"(w1247) -> ()
                n637 = local write "Measurement File_average"(w1249) -> ()
                n638 = local write "Measurement File_up"(w1248) -> ()
                n639 = local write "SaveSweep"(TRUE) -> ()
              }
            }
          }
        }
        n640 = local write "Measurement File"(w1232) -> ()
        n641 = local write "Offset?"(FALSE ("Offset?")) -> ()
        n642 = local write "First?"(TRUE ("First?")) -> ()
      }
      event "Heater On/Off": Value Change {
        n643 = event-data() -> ()  [unwired: 1 in, 6 out]
        n644 = case shown="True" "Heater On/Off" {
          tunnel: w1255 -> [w1260 w1266]
          tunnel: w1254 -> [w1258 w1267]
          tunnel: [w1257 w1265] -> w1253
          frame False {
            n645 = VISA Write(VISA resource name=w1260, write buffer="RANGE,2,0", error in (no error)=w1258) -> (error out=w1257:errorcluster)  [unwired: 2 out]
          }
          frame True {
            n646 = Number To Decimal String(number="Heater Range") -> (decimal integer string=w1263:string)  [unwired: 1 in]
            n647 = Concatenate Strings("RANGE,2," ("write buffer"), w1263) -> (w1261:string)
            n648 = VISA Write(VISA resource name=w1266, write buffer=w1261, error in (no error)=w1267) -> (error out=w1265:errorcluster)  [unwired: 2 out]
          }
        }
      }
      event "Set temperature (K)": Value Change {
        n649 = event-data() -> ()  [unwired: 1 in, 6 out]
        n650 = local read "Set temperature (K)"() -> (w1278:dbl)
        n651 = Number To Fractional String(number=w1278, precision (6)=i16 3) -> (F-format string=w1281:string)  [unwired: 2 in]
        n652 = Select(t="1,  " ("write buffer"), s="Channel B/A", f="2,  " ("write buffer")) -> (s? t:f=w1268:string)
        n653 = Concatenate Strings("SETP " ("write buffer"), w1268, w1281) -> (w1279:string)
        n654 = VISA Write(VISA resource name=w1275, write buffer=w1279, error in (no error)=w1277) -> (error out=w1276:errorcluster)  [unwired: 2 out]
      }
      event "Temp Ramping Rate (K/min)": Value Change {
        n655 = event-data() -> ()  [unwired: 1 in, 6 out]
        n656 = local read "Temp Ramping Rate (K/min)"() -> (w1290:dbl)
        n657 = local read "Channel B/A"() -> (w1284:bool)
        n658 = Number To Fractional String(number=w1290, precision (6)=i16 1) -> (F-format string=w1287:string)  [unwired: 2 in]
        n659 = Select(t="1,1,  " ("write buffer"), s=w1284, f="2,1,  " ("write buffer")) -> (s? t:f=w1282:string)
        n660 = Concatenate Strings("RAMP " ("string"), w1282, w1287) -> (w1294:string)
        n661 = VISA Write(VISA resource name=w1293, write buffer=w1294, error in (no error)=w1292) -> (error out=w1291:errorcluster)  [unwired: 2 out]
      }
      event "Heater Range": Value Change {
        n662 = event-data() -> ()  [unwired: 1 in, 6 out]
        n663 = local read "Heater On/Off"() -> (w1300:bool)
        n664 = case shown="True" w1300 {
          tunnel: w1299 -> [w1301 w1306]
          tunnel: [w1301 w1305] -> w1298
          tunnel: w1296 -> [_ w1304]
          frame False {
          }
          frame True {
            n665 = local read "Heater Range"() -> (w1302:enum16{"Off", "Low", "Medium", "High"})
            n666 = Number To Decimal String(number=w1302) -> (decimal integer string=w1308:string)  [unwired: 1 in]
            n667 = Concatenate Strings("RANGE,2," ("write buffer"), w1308) -> (w1307:string)
            n668 = VISA Write(VISA resource name=w1304, write buffer=w1307, error in (no error)=w1306) -> (error out=w1305:errorcluster)  [unwired: 2 out]
          }
        }
      }
    }
    n669 = Reciprocal(x="Sampling rate (Hz)") -> (1/x=w965:dbl)
    n670 = Multiply(x=w965, y=1000.0) -> (x*y=w963:dbl)
    n671 = Wait Until Next ms Multiple(millisecond multiple=w963) -> ()  [unwired: 1 out]
  }
  n672 = local read "Max Field (T)"() -> (w72:dbl)
  n673 = local read "Min Field (T)"() -> (w74:dbl)
  n674 = local read "dB (T)"() -> (w73:dbl)
  n675 = Divide(x=w72, y=w73) -> (x/y=w75:dbl)
  n676 = for {
    N: w75 -> [_]
    tunnel: w73 -> [w1313]
    tunnel: [w1310] -> w35 mode=indexing
    tunnel: w74 -> [w1311]
    tunnel: [0.0] -> _ mode=indexing
    i -> [w1314]
    n677 = Multiply(x=w1314, y=w1313) -> (x*y=w1312:dbl)
    n678 = Add(x=w1312, y=w1311) -> (x+y=w1310:dbl)
  }
  n679 = Multiply(x=w35, y=0.0) -> (x*y=w32:dbl[])
  n680 = Array Size(array=w32) -> (size(s)=w31:i32)
  n681 = Decrement(x=w31) -> (x-1=w30:i32)
  n682 = local write "B array"(w35) -> ()
  n683 = Array Subset(array=w32, length=w30) -> (w29:dbl[])  [unwired: 1 in]
  n684 = Build Array(w32, w32) -> (w33:dbl[][])
  n685 = local read "Max temperature (K)"() -> (w1:dbl)
  n686 = local read "Min Temperature (K)"() -> (w3:dbl)
  n687 = local write "Averaged I(B)"(w33) -> ()
  n688 = Build Array(w29, w29) -> (w28:dbl[][])
  n689 = Divide(x=w1, y="dt (K)") -> (x/y=w5:dbl)
  n690 = local write "Averaged P(B)"(w28) -> ()
  n691 = local write "Averaged dt"(w28) -> ()
  n692 = for {
    N: w5 -> [_]
    tunnel: "dt (K)" -> [w1319]
    tunnel: [w1316] -> w4 mode=indexing
    tunnel: w3 -> [w1317]
    tunnel: [0.0] -> _ mode=indexing
    i -> [w1320]
    n693 = Multiply(x=w1320, y=w1319) -> (x*y=w1318:dbl)
    n694 = Add(x=w1318, y=w1317) -> (x+y=w1316:dbl)
  }
  "T array" <- w4
  n695 = local read "Lake Shore"() -> (w85:refnum<visa-resource-name>)
  n696 = local read "IV converter"() -> (w101:refnum<visa-resource-name>)
  n697 = local read "Magnetic Field"() -> (w100:refnum<visa-resource-name>)
  n698 = VISA Close(VISA resource name=w101, error in (no error)=w103) -> (error out=w104:errorcluster)
  n699 = VISA Close(VISA resource name=w100, error in (no error)=w104) -> (error out=w102:errorcluster)
  n700 = Release Queue(queue=w108, error in (no error)=w102) -> (error out=w98:errorcluster)  [unwired: 1 in, 2 out]
  n701 = Merge Errors(w98, w97) -> (w99:errorcluster)
  n702 = VISA Close(VISA resource name=w85, error in (no error)=w99) -> (error out=w96:errorcluster)
  n703 = local read "refnum out"() -> (w94:refnum<file>)
  n704 = Close File(refnum=w94, error in=w96) -> (error out=w95:errorcluster)  [unwired: 1 out]
  n705 = call <vilib>:"Simple Error Handler.vi"("error in (no error)"=w95) -> ()  [unwired: 4 in, 5 out]
  "i" <- w65
  "j" <- w65
